vi "LPT-GUI-MIC-ver 5b.vi"() -> ()   [LabVIEW 2019]
uses:
  <vilib>/userDefined/High Color/IMAQdx.ctl
  LabView - DISB Eval SW 2.6/LabView - DISB Eval SW 2.6/Register name.ctl
  <vilib>/Utility/file.llb/Write Delimited Spreadsheet (DBL).vi
  <vilib>/vision/driver/NI_Vision_Acquisition_Software.lvlib
panel:
  in  "LED Resource (write)":refnum<visa-resource-name>="COM3"
  in  "Session In 2":T1="cam6"
  in  "Session In":T1="cam5"
  out "COMMAND1 READ 3":string="LED1 ON\r"
  out "AUT FOCUS STATUS 2":bool
  out "Position (um) 2":dbl(slide) min=0.0 max=100.0 step=0.01 scale=0.0..1500.0
  out "COMMAND 3":string="LED1 OFF"
  out "NUMBER 2":string
  out "Raw Data 2":sgl[](graph)
  out "power sum 2":sgl
  in  "#of steps 3":i32=200
  in  "STAGE START 2":i32
  in  "STAGE STOP 2":i32=20
  out "power sum":sgl
  out "Raw Data":sgl[](graph)
  in  "START CAM TAB":bool
  out "Camera STOP 2":bool
  out "COMMAND1 READ 2":string="LED1 ON\r"
  out "Position (um)":dbl(slide) min=0.0 max=100.0 step=0.01 scale=0.0..1500.0
  out "COMMAND 2":string="LED1 OFF"
  out "NUMBER":string
  in  "#of steps 2":i32=5
  in  "STAGE START":i32
  in  "STAGE STOP":i32=1500
  out "BOROSCOPE END":string
  out "Position (mm)":dbl(slide)=10.0 min=0.0 max=100.0 step=0.01 scale=0.0..20.0 scale format="%.2f"
  out "COMMAND1 READ":string="LED1 ON\r"
  in  "COMMAND 1":string="LED1 OFF"
  out "LASER \nFOCUSED":bool
  in  "INTERACTIVE CONTROLS":T2(radio)
  in  "LQComm resource name":refnum<visa-resource-name>="COM4"
  in  "Analysis Program":T3(radio)
  in  "LIBS Laser Frequency (Hz)":u16=10 min=10 max=1000
  in  "Auto Set\nLaser Frequency":bool
  in  "Acquisition Type":enum32{"RAMAN", "LIBS"}(radio)
  in  "Integration\n Time (ms)":i32=100
  in  "ID spectra":bool
  in  "Number of Scans \nto Auto Acquire":i32=2
  in  "AutoAcquire":bool=TRUE
  out "power setting from LQ":string="POWER=080\r\n"
  out "Power Out":dbl=0.4
  in  "Get Dark?":bool
  in  "Set Power (mW)":i32=80
  in  "Start":bool
  out "Camera STOP":bool
  in  "EXIT INTERACTIVE CONTROL":bool
  in  "ABORT  LOOP":bool
  out "Removed background":dbl[](graph)
  out "LIBS Dark Spectra":dbl[](graph)
  out "Dark Spectra":dbl[](graph)=[1870.0, 1885.0, 1880.0, 1896.0, 1901.0, 1906.0, 1893.0, 1873.0, 1869.0, 1877.0, 1867.0, 1828.0, 1817.0, 1812.0, 1819.0, 1837.0, 1828.0, 1798.0, 1797.0, 1809.0, 1800.0, 1781.0, 1773.0, 1752.0, 1749.0, 1759.0, 1771.0, 1780.0, 1783.0, 1757.0, 1759.0, 1773.0, 1764.0, 1750.0, 1783.0, 1813.0, 1852.0, 1868.0, 1849.0, 1845.0, 1844.0, 1863.0, 1853.0, 1841.0, 1791.0, 1771.0, 1777.0, 1785.0, 1821.0, 1881.0, 1909.0, 1926.0, 1925.0, 1929.0, 1912.0, 1898.0, 1903.0, 1901.0, 1897.0, 1865.0, 1874.0, 1897.0, 1919.0, 1905.0, 1901.0, 1919.0, 1947.0, 1919.0, 1887.0, 1877.0, 1837.0, 1807.0, 1823.0, 1855.0, 1871.0, 1847.0, 1823.0, 1842.0, 1887.0, 1906.0, 1925.0, 1945.0, 1924.0, 1919.0, 1919.0, 1906.0, 1897.0, 1865.0, 1817.0, 1801.0, 1809.0, 1797.0, 1818.0, 1860.0, 1853.0, 1819.0, 1768.0, 1758.0, 1741.0, 1732.0, 1717.0, 1725.0, 1734.0, 1713.0, 1695.0, 1707.0, 1727.0, 1743.0, 1759.0, 1788.0, 1802.0, 1775.0, 1772.0, 1780.0, 1801.0, 1819.0, 1813.0, 1817.0, 1823.0, 1844.0, 1851.0, 1805.0, 1809.0, 1842.0, 1845.0, 1853.0, 1837.0, 1846.0, 1837.0, 1853.0, 1862.0, 1881.0, 1901.0, 1874.0, 1861.0, 1892.0, 1876.0, 1872.0, 1855.0, 1846.0, 1860.0, 1861.0, 1887.0, 1887.0, 1883.0, 1897.0, 1897.0, 1903.0, 1911.0, 1901.0, 1880.0, 1871.0, 1855.0, 1879.0, 1860.0, 1871.0, 1880.0, 1879.0, 1858.0, 1855.0, 1837.0, 1837.0, 1823.0, 1828.0, 1807.0, 1821.0, 1882.0, 1890.0, 1893.0, 1860.0, 1832.0, 1812.0, 1813.0, 1842.0, 1852.0, 1849.0, 1851.0, 1835.0, 1849.0, 1885.0, 1924.0, 1930.0, 1930.0, 1925.0, 1892.0, 1897.0, 1903.0, 1900.0, 1912.0, 1917.0, 1946.0, 1947.0, 1927.0, 1896.0, 1881.0, 1896.0, 1874.0, 1873.0, 1876.0, 1898.0, 1899.0, 1885.0, 1892.0, 1897.0, 1896.0, 1896.0, 1878.0, 1870.0, 1860.0, 1853.0, 1867.0, 1855.0, 1839.0, 1839.0, 1849.0, 1853.0, 1846.0, 1829.0, 1817.0, 1828.0, 1823.0, 1860.0, 1881.0, 1863.0, 1885.0, 1860.0, 1833.0, 1846.0, 1832.0, 1844.0, 1813.0, 1815.0, 1837.0, 1833.0, 1837.0, 1828.0, 1829.0, 1844.0, 1840.0, 1849.0, 1844.0, 1812.0, 1815.0, 1801.0, 1814.0, 1815.0, 1837.0, 1832.0, 1840.0, 1812.0, 1797.0, 1815.0, 1862.0, 1899.0, 1906.0, 1905.0, 1885.0, 1868.0, 1861.0, 1845.0, 1832.0, 1797.0, 1803.0, 1791.0, 1791.0, 1784.0, 1801.0, 1786.0, 1768.0, 1765.0, 1759.0, 1745.0, 1743.0, 1774.0, 1813.0, 1820.0, 1855.0, 1881.0, 1881.0, 1887.0, 1876.0, 1870.0, 1864.0, 1897.0, 1897.0, 1887.0, 1873.0, 1853.0, 1833.0, 1807.0, 1802.0, 1791.0, 1823.0, 1828.0, 1812.0, 1850.0, 1853.0, 1846.0, 1839.0, 1837.0, 1852.0, 1849.0, 1828.0, 1848.0, 1864.0, 1860.0, 1864.0, 1846.0, 1829.0, 1837.0, 1835.0, 1819.0, 1807.0, 1812.0, 1805.0, 1789.0, 1798.0, 1802.0, 1818.0, 1783.0, 1796.0, 1804.0, 1837.0, 1876.0, 1935.0, 1994.0, 2007.0, 1969.0, 1961.0, 1938.0, 1917.0, 1908.0, 1901.0, 1885.0, 1911.0, 1930.0, 1929.0, 1945.0, 1919.0, 1899.0, 1870.0, 1855.0, 1825.0, 1814.0, 1817.0, 1797.0, 1803.0, 1791.0, 1789.0, 1768.0, 1734.0, 1757.0, 1757.0, 1737.0, 1752.0, 1773.0, 1768.0, 1761.0, 1759.0, 1784.0, 1783.0, 1803.0, 1791.0, 1791.0, 1796.0, 1791.0, 1781.0, 1773.0, 1761.0, 1780.0, 1791.0, 1780.0, 1773.0, 1759.0, 1757.0, 1769.0, 1773.0, 1768.0, 1780.0, 1780.0, 1782.0, 1807.0, 1805.0, 1789.0, 1807.0, 1836.0, 1823.0, 1839.0, 1873.0, 1873.0, 1893.0, 1892.0, 1868.0, 1876.0, 1887.0, 1896.0, 1899.0, 1892.0, 1867.0, 1851.0, 1848.0, 1839.0, 1865.0, 1866.0, 1849.0, 1834.0, 1839.0, 1862.0, 1861.0, 1851.0, 1839.0, 1849.0, 1847.0, 1828.0, 1789.0, 1769.0, 1787.0, 1779.0, 1797.0, 1816.0, 1846.0, 1855.0, 1855.0, 1863.0, 1869.0, 1885.0, 1892.0, 1901.0, 1946.0, 1913.0, 1880.0, 1896.0, 1901.0, 1877.0, 1881.0, 1878.0, 1855.0, 1845.0, 1832.0, 1799.0, 1769.0, 1757.0, 1781.0, 1762.0, 1735.0, 1714.0, 1733.0, 1757.0, 1773.0, 1773.0, 1783.0, 1778.0, 1768.0, 1764.0, 1765.0, 1753.0, 1738.0, 1759.0, 1781.0, 1789.0, 1800.0, 1799.0, 1796.0, 1785.0, 1771.0, 1727.0, 1700.0, 1723.0, 1711.0, 1716.0, 1738.0, 1773.0, 1781.0, 1769.0, 1778.0, 1768.0, 1771.0, 1775.0, 1781.0, 1768.0, 1744.0, 1739.0, 1732.0, 1716.0, 1695.0, 1689.0, 1695.0, 1679.0, 1695.0, 1692.0, 1717.0, 1718.0, 1721.0, 1695.0, 1679.0, 1677.0, 1675.0, 1678.0, 1679.0, 1682.0, 1689.0, 1684.0, 1711.0, 1711.0, 1721.0, 1727.0, 1727.0, 1723.0, 1707.0, 1732.0, 1721.0, 1724.0, 1700.0, 1692.0, 1685.0, 1693.0, 1695.0, 1705.0, 1694.0, 1700.0, 1722.0, 1714.0, 1719.0, 1723.0, 1711.0, 1721.0, 1746.0, 1775.0, 1756.0, 1704.0, 1692.0, 1721.0, 1725.0, 1718.0, 1712.0, 1725.0, 1732.0, 1741.0, 1745.0, 1773.0, 1784.0, 1782.0, 1785.0, 1800.0, 1800.0, 1785.0, 1757.0, 1759.0, 1718.0, 1725.0, 1725.0, 1736.0, 1770.0, 1802.0, 1808.0, 1801.0, 1809.0, 1812.0, 1794.0, 1823.0, 1842.0, 1839.0, 1849.0, 1823.0, 1832.0, 1823.0, 1801.0, 1812.0, 1832.0, 1823.0, 1810.0, 1810.0, 1796.0, 1816.0, 1797.0, 1853.0, 1871.0, 1883.0, 1887.0, 1902.0, 1884.0, 1869.0, 1853.0, 1832.0, 1823.0, 1812.0, 1821.0, 1823.0, 1832.0, 1821.0, 1823.0, 1809.0, 1784.0, 1752.0, 1732.0, 1727.0, 1721.0, 1709.0, 1735.0, 1727.0, 1725.0, 1707.0, 1698.0, 1682.0, 1689.0, 1714.0, 1716.0, 1707.0, 1709.0, 1714.0, 1725.0, 1727.0, 1738.0, 1725.0, 1741.0, 1739.0, 1701.0, 1733.0, 1727.0, 1717.0, 1718.0, 1752.0, 1775.0, 1775.0, 1784.0, 1802.0, 1771.0, 1759.0, 1750.0, 1724.0, 1721.0, 1711.0, 1689.0, 1677.0, 1666.0, 1686.0, 1698.0, 1711.0, 1750.0, 1741.0, 1756.0, 1771.0, 1768.0, 1787.0, 1796.0, 1807.0, 1790.0, 1809.0, 1842.0, 1832.0, 1807.0, 1805.0, 1805.0, 1764.0, 1789.0, 1785.0, 1669.0, 1625.0, 1631.0, 1637.0, 1642.0, 1599.0, 1605.0, 1579.0, 1592.0, 1576.0, 1590.0, 1604.0, 1615.0, 1659.0, 1672.0, 1669.0, 1689.0, 1672.0, 1672.0, 1701.0, 1716.0, 1741.0, 1730.0, 1719.0, 1711.0, 1695.0, 1706.0, 1721.0, 1770.0, 1796.0, 1797.0, 1768.0, 1765.0, 1781.0, 1765.0, 1759.0, 1749.0, 1781.0, 1786.0, 1804.0, 1796.0, 1777.0, 1768.0, 1772.0, 1778.0, 1821.0, 1821.0, 1823.0, 1837.0, 1845.0, 1829.0, 1849.0, 1833.0, 1832.0, 1797.0, 1771.0, 1764.0, 1791.0, 1786.0, 1764.0, 1743.0, 1730.0, 1752.0, 1746.0, 1741.0, 1741.0, 1748.0, 1757.0, 1784.0, 1775.0, 1777.0, 1796.0, 1810.0, 1799.0, 1814.0, 1768.0, 1773.0, 1780.0, 1765.0, 1764.0, 1769.0, 1748.0, 1732.0, 1709.0, 1706.0, 1695.0, 1679.0, 1675.0, 1669.0, 1679.0, 1707.0, 1721.0, 1711.0, 1704.0, 1701.0, 1700.0, 1695.0, 1695.0, 1668.0, 1692.0, 1711.0, 1725.0, 1716.0, 1693.0, 1700.0, 1720.0, 1704.0, 1711.0, 1716.0, 1725.0, 1721.0, 1706.0, 1700.0, 1706.0, 1717.0, 1732.0, 1717.0, 1721.0, 1695.0, 1695.0, 1698.0, 1688.0, 1689.0, 1691.0, 1687.0, 1709.0, 1717.0, 1732.0, 1725.0, 1668.0, 1672.0, 1673.0, 1681.0, 1688.0, 1707.0, 1725.0, 1739.0, 1716.0, 1641.0, 1636.0, 1642.0, 1655.0, 1663.0, 1675.0, 1675.0, 1700.0, 1730.0, 1764.0, 1803.0, 1816.0, 1820.0, 1807.0, 1791.0, 1759.0, 1753.0, 1761.0, 1759.0, 1753.0, 1744.0, 1775.0, 1781.0, 1768.0, 1753.0, 1741.0, 1721.0, 1725.0, 1743.0, 1748.0, 1747.0, 1771.0, 1775.0, 1771.0, 1756.0, 1753.0, 1709.0, 1716.0, 1704.0, 1734.0, 1737.0, 1725.0, 1721.0, 1724.0, 1716.0, 1732.0, 1744.0, 1775.0, 1751.0, 1706.0, 1704.0, 1716.0, 1709.0, 1717.0, 1741.0, 1761.0, 1764.0, 1781.0, 1791.0, 1764.0, 1746.0, 1732.0, 1734.0, 1727.0, 1716.0, 1700.0, 1686.0, 1684.0, 1686.0, 1707.0, 1732.0, 1727.0, 1738.0, 1716.0, 1705.0, 1709.0, 1707.0, 1700.0, 1698.0, 1698.0, 1716.0, 1723.0, 1705.0, 1717.0, 1689.0, 1690.0, 1687.0, 1684.0, 1719.0, 1717.0, 1714.0, 1690.0, 1668.0, 1663.0, 1675.0, 1677.0, 1684.0, 1673.0, 1668.0, 1679.0, 1695.0, 1706.0, 1735.0, 1748.0, 1747.0, 1759.0, 1764.0, 1757.0, 1732.0, 1750.0, 1781.0, 1764.0, 1764.0, 1749.0, 1754.0, 1756.0, 1741.0, 1739.0, 1741.0, 1714.0, 1733.0, 1762.0, 1759.0, 1768.0, 1775.0, 1768.0, 1759.0, 1768.0, 1750.0, 1739.0, 1757.0, 1757.0, 1727.0, 1748.0, 1723.0, 1725.0, 1709.0, 1709.0, 1709.0, 1731.0, 1734.0, 1748.0, 1759.0, 1757.0, 1759.0, 1752.0, 1741.0, 1755.0, 1787.0, 1791.0, 1820.0, 1840.0, 1860.0, 1873.0, 1874.0, 1865.0, 1876.0, 1876.0, 1844.0, 1844.0, 1849.0, 1862.0, 1832.0, 1828.0, 1842.0, 1832.0, 1796.0, 1788.0, 1751.0, 1764.0, 1756.0, 1746.0, 1739.0, 1733.0, 1726.0, 1705.0, 1700.0, 1723.0, 1725.0, 1725.0, 1739.0, 1759.0, 1777.0, 1771.0, 1759.0, 1771.0, 1765.0, 1753.0, 1725.0, 1684.0, 1647.0, 1636.0, 1652.0, 1657.0, 1669.0, 1672.0, 1677.0, 1653.0, 1672.0, 1657.0, 1661.0, 1660.0, 1676.0, 1704.0, 1707.0, 1729.0, 1757.0, 1796.0, 1797.0, 1802.0, 1797.0, 1807.0, 1844.0, 1835.0, 1794.0, 1791.0, 1796.0, 1801.0, 1789.0, 1791.0, 1782.0, 1768.0, 1739.0, 1723.0, 1736.0, 1732.0, 1737.0, 1733.0, 1727.0, 1707.0, 1677.0, 1695.0, 1704.0, 1714.0, 1690.0, 1657.0, 1661.0, 1669.0, 1656.0, 1652.0, 1611.0, 1595.0, 1549.0, 1562.0, 1596.0, 1610.0, 1573.0, 1576.0, 1577.0, 1567.0, 1573.0, 1605.0, 1592.0, 1622.0, 1621.0, 1609.0, 1599.0, 1606.0, 1581.0, 1565.0, 1567.0, 1589.0, 1610.0, 1607.0, 1608.0, 1643.0, 1647.0, 1668.0, 1691.0, 1675.0, 1641.0, 1647.0, 1640.0, 1622.0, 1621.0, 1588.0, 1602.0, 1622.0, 1611.0, 1599.0, 1602.0, 1640.0, 1643.0, 1647.0, 1629.0, 1577.0, 1547.0, 1554.0, 1551.0, 1540.0, 1561.0, 1561.0, 1576.0, 1614.0, 1674.0, 1707.0, 1717.0, 1736.0, 1735.0, 1743.0, 1738.0, 1727.0, 1735.0, 1721.0, 1721.0, 1687.0, 1707.0, 1709.0, 1748.0, 1743.0, 1743.0, 1753.0, 1769.0, 1759.0, 1765.0, 1737.0, 1727.0, 1711.0, 1679.0, 1672.0, 1686.0, 1672.0, 1668.0, 1660.0, 1645.0, 1669.0, 1688.0, 1685.0, 1679.0, 1721.0, 1739.0, 1712.0, 1681.0, 1650.0, 1653.0, 1661.0, 1663.0, 1663.0, 1668.0, 1672.0, 1704.0, 1714.0, 1721.0, 1718.0, 1814.0, 1797.0, 1759.0, 1754.0, 1743.0, 1762.0, 1748.0, 1768.0, 1741.0, 1690.0, 1707.0, 1717.0, 1739.0, 1768.0, 1727.0, 1682.0, 1650.0, 1681.0, 1701.0, 1727.0, 1695.0, 1676.0, 1673.0, 1669.0, 1677.0, 1663.0, 1674.0, 1690.0, 1687.0, 1668.0, 1690.0, 1725.0, 1689.0, 1647.0, 1627.0, 1615.0, 1647.0, 1656.0, 1631.0, 1625.0, 1618.0, 1609.0, 1608.0, 1636.0, 1674.0, 1720.0, 1738.0, 1745.0, 1736.0, 1738.0, 1762.0, 1781.0, 1776.0, 1794.0, 1798.0, 1757.0, 1741.0, 1717.0, 1711.0, 1725.0, 1727.0, 1732.0, 1730.0, 1701.0, 1700.0, 1657.0, 1652.0, 1668.0, 1653.0, 1621.0, 1629.0, 1611.0, 1615.0, 1608.0, 1583.0, 1599.0, 1636.0, 1668.0, 1684.0, 1705.0, 1701.0, 1725.0, 1752.0, 1746.0, 1749.0, 1727.0, 1755.0, 1746.0, 1749.0, 1764.0, 1752.0, 1739.0, 1768.0, 1757.0, 1711.0, 1677.0, 1657.0, 1653.0, 1661.0, 1647.0, 1618.0, 1620.0, 1649.0, 1675.0, 1668.0, 1672.0, 1679.0, 1656.0, 1669.0, 1674.0, 1700.0, 1705.0, 1704.0, 1700.0, 1705.0, 1718.0, 1711.0, 1705.0, 1701.0, 1718.0, 1713.0, 1736.0, 1752.0, 1748.0, 1732.0, 1750.0, 1765.0, 1741.0, 1723.0, 1725.0, 1705.0, 1676.0, 1641.0, 1636.0, 1631.0, 1631.0, 1656.0, 1663.0, 1666.0, 1668.0, 1669.0, 1629.0, 1647.0, 1610.0, 1551.0, 1494.0, 1483.0, 1465.0, 1476.0, 1487.0, 1512.0, 1553.0, 1573.0, 1556.0, 1501.0, 1503.0, 1531.0, 1567.0, 1624.0, 1663.0, 1661.0, 1657.0, 1645.0, 1616.0, 1621.0, 1594.0, 1529.0, 1503.0, 1490.0, 1476.0, 1501.0, 1501.0, 1517.0, 1527.0, 1558.0, 1567.0, 1586.0, 1556.0, 1547.0, 1548.0, 1551.0, 1497.0, 1439.0, 1428.0, 1459.0, 1516.0, 1563.0, 1558.0, 1609.0, 1657.0, 1693.0, 1734.0, 1753.0, 1765.0, 1773.0, 1796.0, 1800.0, 1815.0, 1821.0, 1851.0, 1855.0, 1844.0, 1844.0, 1846.0, 1850.0, 1833.0, 1786.0, 1791.0, 1791.0, 1789.0, 1798.0, 1797.0, 1802.0, 1809.0, 1819.0, 1820.0, 1816.0, 1796.0, 1804.0, 1804.0, 1786.0, 1794.0, 1753.0, 1764.0, 1800.0, 1811.0, 1809.0, 1816.0, 1785.0, 1765.0, 1735.0, 1687.0, 1672.0, 1661.0, 1621.0, 1583.0, 1482.0, 1444.0, 1451.0, 1471.0, 1500.0, 1541.0, 1530.0, 1541.0, 1540.0, 1581.0, 1605.0, 1649.0, 1659.0, 1660.0, 1654.0, 1672.0, 1668.0, 1691.0, 1692.0, 1693.0, 1672.0, 1674.0, 1693.0, 1707.0, 1735.0, 1759.0, 1758.0, 1752.0, 1759.0, 1763.0, 1764.0, 1757.0, 1741.0, 1727.0, 1727.0, 1720.0, 1738.0, 1733.0, 1735.0, 1725.0, 1743.0, 1746.0, 1753.0, 1752.0, 1750.0, 1738.0, 1755.0, 1746.0, 1764.0, 1787.0, 1775.0, 1748.0, 1725.0, 1725.0, 1759.0, 1775.0, 1791.0, 1804.0, 1823.0, 1842.0, 1839.0, 1846.0, 1807.0, 1812.0, 1835.0, 1819.0, 1837.0, 1799.0, 1769.0, 1765.0, 1759.0, 1781.0, 1768.0, 1727.0, 1689.0, 1672.0, 1636.0, 1629.0, 1629.0, 1647.0, 1645.0, 1641.0, 1640.0, 1658.0, 1640.0, 1642.0, 1645.0, 1672.0, 1700.0, 1701.0, 1688.0, 1709.0, 1727.0, 1732.0, 1759.0, 1754.0, 1765.0, 1746.0, 1727.0, 1725.0, 1759.0, 1752.0, 1753.0, 1768.0, 1759.0, 1764.0, 1759.0, 1773.0, 1794.0, 1796.0, 1791.0, 1812.0, 1805.0, 1810.0, 1801.0, 1791.0, 1782.0, 1787.0, 1775.0, 1775.0, 1775.0, 1780.0, 1783.0, 1807.0, 1815.0, 1821.0, 1800.0, 1823.0, 1819.0, 1801.0, 1779.0, 1773.0, 1780.0, 1788.0, 1804.0, 1800.0, 1789.0, 1757.0, 1743.0, 1727.0, 1721.0, 1732.0, 1720.0, 1681.0, 1681.0, 1701.0, 1684.0, 1650.0, 1645.0, 1656.0, 1684.0, 1686.0, 1677.0, 1691.0, 1685.0, 1700.0, 1721.0, 1741.0, 1758.0, 1749.0, 1733.0, 1695.0, 1701.0, 1687.0, 1712.0, 1721.0, 1738.0, 1759.0, 1796.0, 1823.0, 1849.0, 1860.0, 1868.0, 1855.0, 1848.0, 1855.0, 1844.0, 1809.0, 1810.0, 1832.0, 1807.0, 1800.0, 1829.0, 1837.0, 1823.0, 1805.0, 1828.0, 1848.0, 1855.0, 1838.0, 1807.0, 1804.0, 1802.0, 1806.0, 1823.0, 1807.0, 1807.0, 1816.0, 1844.0, 1862.0, 1879.0, 1882.0, 1877.0, 1875.0, 1897.0, 1855.0, 1837.0, 1835.0, 1817.0, 1810.0, 1789.0, 1751.0, 1741.0, 1723.0, 1722.0, 1718.0, 1752.0, 1773.0, 1768.0, 1781.0, 1739.0, 1709.0, 1693.0, 1709.0, 1722.0, 1727.0, 1724.0, 1749.0, 1725.0, 1748.0, 1758.0, 1769.0, 1778.0, 1771.0, 1770.0, 1745.0, 1736.0, 1771.0, 1768.0, 1748.0, 1756.0, 1773.0, 1748.0, 1754.0, 1772.0, 1804.0, 1803.0, 1805.0, 1768.0, 1750.0, 1764.0, 1741.0, 1748.0, 1727.0, 1707.0, 1707.0, 1737.0, 1721.0, 1717.0, 1722.0, 1720.0, 1734.0, 1750.0, 1725.0, 1725.0, 1736.0, 1691.0, 1681.0, 1689.0, 1677.0, 1675.0, 1707.0, 1712.0, 1704.0, 1684.0, 1679.0, 1677.0, 1683.0, 1663.0, 1636.0, 1640.0, 1640.0, 1657.0, 1669.0, 1677.0, 1704.0, 1727.0, 1769.0, 1741.0, 1749.0, 1759.0, 1757.0, 1762.0, 1750.0, 1749.0, 1759.0, 1759.0, 1775.0, 1773.0, 1823.0, 1815.0, 1807.0, 1821.0, 1813.0, 1805.0, 1817.0, 1813.0, 1821.0, 1807.0, 1803.0, 1805.0, 1821.0, 1828.0, 1817.0, 1805.0, 1802.0, 1791.0, 1776.0, 1768.0, 1770.0, 1755.0, 1738.0, 1764.0, 1757.0, 1751.0, 1759.0, 1762.0, 1786.0, 1771.0, 1775.0, 1801.0, 1807.0, 1797.0, 1786.0, 1855.0, 1879.0, 1878.0, 1852.0, 1834.0, 1845.0, 1849.0, 1869.0, 1865.0, 1855.0, 1885.0, 1885.0, 1860.0, 1812.0, 1803.0, 1790.0, 1784.0, 1773.0, 1769.0, 1751.0, 1739.0, 1721.0, 1749.0, 1738.0, 1742.0, 1743.0, 1718.0, 1687.0, 1685.0, 1700.0, 1724.0, 1753.0, 1746.0, 1745.0, 1781.0, 1810.0, 1812.0, 1823.0, 1805.0, 1821.0, 1820.0, 1790.0, 1780.0, 1791.0, 1798.0, 1804.0, 1837.0, 1869.0, 1871.0, 1884.0, 1887.0, 1887.0, 1906.0, 1906.0, 1917.0, 1897.0, 1870.0, 1892.0, 1885.0, 1866.0, 1855.0, 1861.0, 1840.0, 1849.0, 1860.0, 1853.0, 1823.0, 1832.0, 1855.0, 1853.0, 1853.0, 1836.0, 1832.0, 1829.0, 1835.0, 1819.0, 1805.0, 1797.0, 1770.0, 1768.0, 1769.0, 1796.0, 1759.0, 1766.0, 1780.0, 1822.0, 1839.0, 1876.0, 1892.0, 1878.0, 1865.0, 1846.0, 1844.0, 1817.0, 1828.0, 1821.0, 1807.0, 1801.0, 1771.0, 1807.0, 1783.0, 1789.0, 1778.0, 1787.0, 1780.0, 1765.0, 1768.0, 1773.0, 1777.0, 1773.0, 1775.0, 1781.0, 1771.0, 1777.0, 1789.0, 1802.0, 1818.0, 1823.0, 1805.0, 1804.0, 1801.0, 1802.0, 1828.0, 1791.0, 1784.0, 1765.0, 1756.0, 1748.0, 1727.0, 1712.0, 1714.0, 1749.0, 1775.0, 1789.0, 1780.0, 1781.0, 1756.0, 1755.0, 1759.0, 1771.0, 1759.0, 1755.0, 1748.0, 1748.0, 1743.0, 1708.0, 1707.0, 1704.0, 1672.0, 1650.0, 1631.0, 1650.0, 1652.0, 1652.0, 1660.0, 1669.0, 1685.0, 1713.0, 1711.0, 1692.0, 1734.0, 1753.0, 1753.0, 1759.0, 1727.0, 1736.0, 1771.0, 1786.0, 1789.0, 1764.0, 1732.0, 1736.0, 1737.0, 1736.0, 1736.0, 1761.0, 1768.0, 1759.0, 1768.0, 1748.0, 1716.0, 1723.0, 1733.0, 1725.0, 1727.0, 1738.0, 1727.0, 1732.0, 1735.0, 1756.0, 1791.0, 1791.0, 1796.0, 1832.0, 1865.0, 1885.0, 1884.0, 1885.0, 1873.0, 1878.0, 1855.0, 1821.0, 1812.0, 1819.0, 1823.0, 1809.0, 1816.0, 1813.0, 1808.0, 1803.0, 1807.0, 1795.0, 1805.0, 1823.0, 1821.0, 1839.0, 1844.0, 1861.0, 1861.0, 1892.0, 1913.0, 1919.0, 1885.0, 1885.0, 1885.0, 1869.0, 1861.0, 1871.0, 1885.0, 1930.0, 1929.0, 1883.0, 1887.0, 1877.0, 1865.0, 1855.0, 1851.0, 1835.0, 1821.0, 1808.0, 1759.0, 1773.0, 1783.0, 1773.0, 1786.0, 1781.0, 1768.0, 1776.0, 1757.0, 1785.0, 1802.0, 1797.0, 1796.0, 1805.0, 1808.0, 1800.0, 1798.0, 1821.0, 1832.0, 1799.0, 1795.0, 1800.0, 1813.0, 1823.0, 1842.0, 1887.0, 1909.0, 1909.0, 1908.0, 1893.0, 1865.0, 1855.0, 1832.0, 1828.0, 1805.0, 1819.0, 1832.0, 1818.0, 1820.0, 1805.0, 1784.0, 1780.0, 1785.0, 1783.0, 1789.0, 1752.0, 1740.0, 1711.0, 1721.0, 1736.0, 1732.0, 1727.0, 1738.0, 1756.0, 1804.0, 1817.0, 1832.0, 1846.0, 1853.0, 1833.0, 1817.0, 1807.0, 1776.0, 1775.0, 1757.0, 1750.0, 1745.0, 1771.0, 1778.0, 1800.0, 1805.0, 1781.0, 1797.0, 1796.0, 1789.0, 1778.0, 1759.0, 1744.0, 1751.0, 1755.0, 1762.0, 1737.0, 1725.0, 1746.0, 1769.0, 1809.0, 1815.0, 1813.0, 1786.0, 1769.0, 1768.0, 1770.0, 1764.0, 1765.0, 1768.0, 1755.0, 1736.0, 1759.0, 0.0, 0.0, 0.0, 0.0, 0.0]
  out "STATUS":string="INITIALIZING LIBS"
  in  "STAGE STOP A":i32=19 min=10 max=19 format="%.2f"
  in  "STAGE START A":i32=1 min=1 max=10 format="%.2f"
  in  "#of steps A":i32=18 min=2 max=100
  in  "AUT FOCUS":bool
  out "Spectrum":cluster{dbl[], "Dark Array":dbl[]}(graph)
  out "msPerClock":dbl
  in  "SPI clock frequency [Hz]":u32
  in  "*Cal coef":dbl[](array[numeric])=[0.0] format="%.7e"
  in  "*Wavelength axis":dbl[](array[numeric]) format="%.7e"
  in  "Pixel axis":u16[](array[numeric])
  out "Dark spectrum":dbl[](array[numeric])
  out "Ref spectrum":dbl[](array[numeric])
  in  "*Production mode":u16 format="%x"
  in  "*Sensor ctrl":u16
  in  "Skipping start read buffer":u16 max=4096
  in  "Skipping end read buffer":u16=17 min=17 max=4096
  in  "*Last pixel of interest":u16=17 min=17 max=4096
  in  "*First pixel of interest":u16 max=4096
  out "*FW - Reserved":u16
  out "*FW - Variant":u16
  out "*FW - Revision":u16
  out "*Spectrometer SN":u16
  out "Average in progress":bool
  in  "*Auto trig":bool=TRUE
  in  "*Averaging in HW":u16=1
  in  "*Data ready threshold":u16=1
  in  "*MPP mode change":u16
  out "Debug":u16
  out "*ADC offset [counts]":u16
  out "*ADC gain [counts]":u16
  out "Trigger delay MSB":u16
  out "Trigger delay LSB":u16
  out "Pixels ready":u16
  out "*Temperature  [counts] \n(12 bit ADC)":dbl
  out "Sensor exp time MSB":u16
  out "Sensor exp time LSB":u16
  out "*Calib data chars":u16
  out "*Pixels per image":u16
  out "*Detector type":u16
  out "*FW version":u16
  out "*HW version":u16
  out "*PCB SN":u16
  in  "Zero Dark LIBS":dbl[](array[numeric])
  in  "Data\\Dark":bool
  out "MaxPosition":dbl=500.0 format="%#_2f"
  out "max value":sgl=3651732.0
  in  "Zero Dark":dbl[](array[numeric])
  in  "Channel Settings":T4(array[cluster])=[{"Integration Time (msec)"=80, "Xtrate"=1, "Averaging"=5, "Smoothing"=4, "C1"=0.0, "C2"=0.0, "C3"=0.0, "C4"=0.0, "Digitizer Bits"=enum."12"}, {"Integration Time (msec)"=80, "Xtrate"=1, "Averaging"=5, "Smoothing"=4, "C1"=0.0, "C2"=0.0, "C3"=0.0, "C4"=0.0, "Digitizer Bits"=enum."12"}, {"Integration Time (msec)"=80, "Xtrate"=1, "Averaging"=5, "Smoothing"=4, "C1"=0.0, "C2"=0.0, "C3"=0.0, "C4"=0.0, "Digitizer Bits"=enum."12"}, {"Integration Time (msec)"=80, "Xtrate"=1, "Averaging"=5, "Smoothing"=4, "C1"=0.0, "C2"=0.0, "C3"=0.0, "C4"=0.0, "Digitizer Bits"=enum."12"}, {"Integration Time (msec)"=80, "Xtrate"=1, "Averaging"=5, "Smoothing"=4, "C1"=0.0, "C2"=0.0, "C3"=0.0, "C4"=0.0, "Digitizer Bits"=enum."12"}, {"Integration Time (msec)"=80, "Xtrate"=1, "Averaging"=5, "Smoothing"=4, "C1"=0.0, "C2"=0.0, "C3"=0.0, "C4"=0.0, "Digitizer Bits"=enum."12"}, {"Integration Time (msec)"=80, "Xtrate"=1, "Averaging"=5, "Smoothing"=4, "C1"=0.0, "C2"=0.0, "C3"=0.0, "C4"=0.0, "Digitizer Bits"=enum."12"}, {"Integration Time (msec)"=80, "Xtrate"=1, "Averaging"=5, "Smoothing"=4, "C1"=0.0, "C2"=0.0, "C3"=0.0, "C4"=0.0, "Digitizer Bits"=enum."12"}] caption="Spectrometer Configs" {"C4" format="%#.15f"; "C3" format="%#.15f"; "C2" format="%#.15f"; "C1" format="%#.15f"; "Smoothing" min=0 max=4 step=1; "Averaging" min=1 max=10000 step=1; "Xtrate" min=1 max=3; "Integration Time (msec)" min=1 max=2000}
  out "output\ncluster":T5={"Integration Time (ms)"=80, "Digitizer Clock Rate Setting"=3, "Number of Scans to Average"=1, "Optical Smoothing Level"=0, 0.096038248763, 3.43035e-07, -1.607e-09, -1.607e-09, 12}
  in  "RAMAN Spectometer\n Parameters":T6={"Integration Time (ms)"=80, "Digitizer Clock Rate Setting"=3, "Number of Scans to Average"=1, "Optical Smoothing Level"=0, "C1"=0.096038248763, "C2"=3.43035e-07, "C3"=536.3, "C4"=-1.607e-09, 12}
  in  "Tab Control":enum32{"Visible", "Fluorescence"}(tab)
  out "Visible Image":T7(plugin-control)
  out "Fluorescence Image":T7(plugin-control)
  in  "MOVE SPECTROMETER":bool
  out "AUT FOCUS STATUS":bool
  in  "Set End Position (um)":dbl(slide) scale=0.0..1500.0
  out "LED 2 STATUS":bool
  in  "LED 2":bool
  in  "LED 1":bool
  out "LED 1 STATUS":bool
  # "Laser and Plasma RAMAN/LIBS Acquisition Software"
  # "INITIAL SETTINGS"
  # "Raman Laser Settings"
  # "LIBS Laser Settings"
  # "LQC"
  # "LED"
  # "AUTO FOCUS SETTINGS"
  # "AUTO FOCUS RESULTS"
  # "V5b"
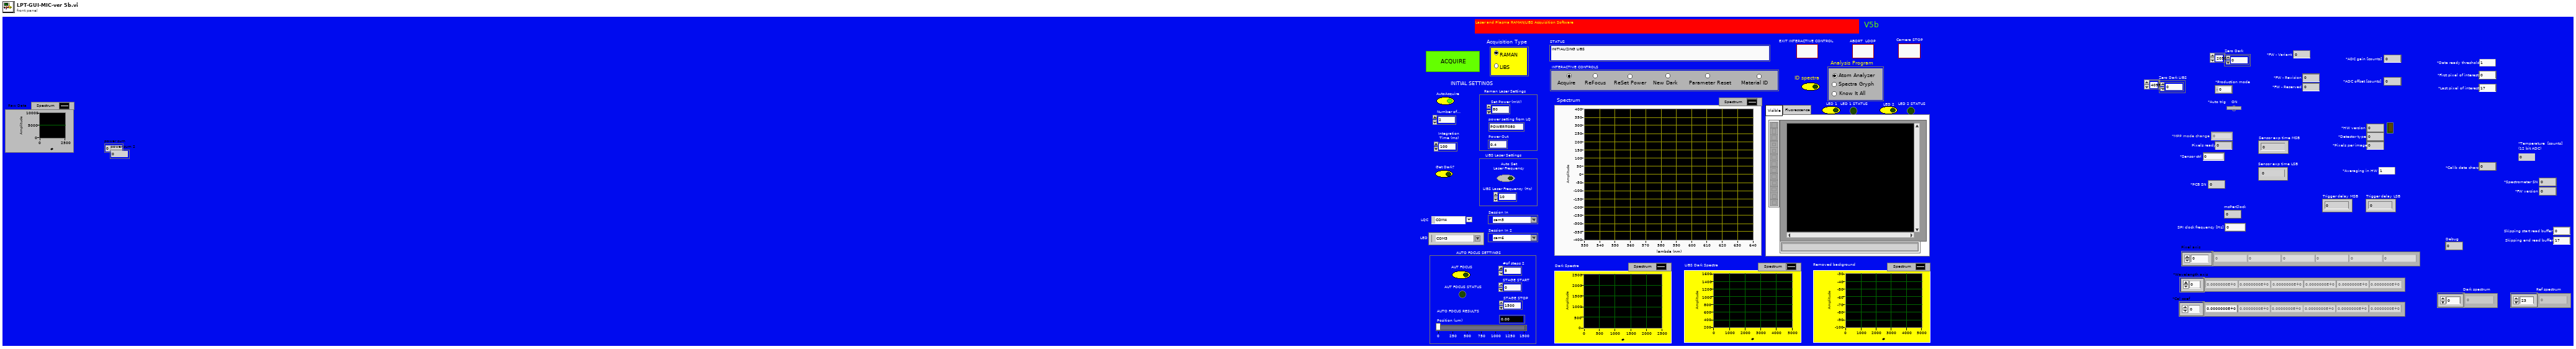
[diagram p1: front panel]
types:
  T1 = typedef "IMAQdx.ctl" = refnum<k21>
  T2 = enum32{"Acquire", "ReFocus", "ReSet Power", "New Dark", "Parameter Reset", "Material ID", "Do Nothing"}
  T3 = enum32{"Atom Analyzer", "Spectra Gryph", "Know It All"}
  T4 = cluster{"Integration Time (msec)":i32, "Xtrate":i32, "Averaging":i32, "Smoothing":i32, "C1":dbl, "C2":dbl, "C3":dbl, "C4":dbl, "Digitizer Bits":enum8{"12", "14", "16"}}[]
  T5 = cluster{"Integration Time (ms)":i32, "Digitizer Clock Rate Setting":i32, "Number of Scans to Average":i32, "Optical Smoothing Level":i32, dbl, dbl, dbl, dbl, i32}
  T6 = typedef "Control 1.ctl" = cluster{"Integration Time (ms)":i32, "Digitizer Clock Rate Setting":i32, "Number of Scans to Average":i32, "Optical Smoothing Level":i32, "C1":dbl, "C2":dbl, "C3":dbl, "C4":dbl, i32}
  T7 = typedef "IMAQ Image.ctl" = refnum<image>
  T8 = typedef "Register name.ctl" = enum8{"Serial number", "HW version", "FW version", "Detector type", "Pixel per image", "Calib data chars", "Calib data", "Sensor ctrl", "Sensor exp time LSB", "Sensor exp time MSB", "Temperature", "Pixel ready", "Trigger delay LSB", "Trigger delay MSB", "ADC PGA", "ADC offset", "Permanent storage", "MPP mode change", "DATA READY THRESHOLD", "IMAGES_TO_AVERAGE", "AVG_CONTROL", "SPECTROMETER SN", "SKIPPING_START", "SKIPPING_END", "debug", "Production mode"}
  T9 = enum8{"Enabled", "Disabled", "Disabled and Grayed Out"}
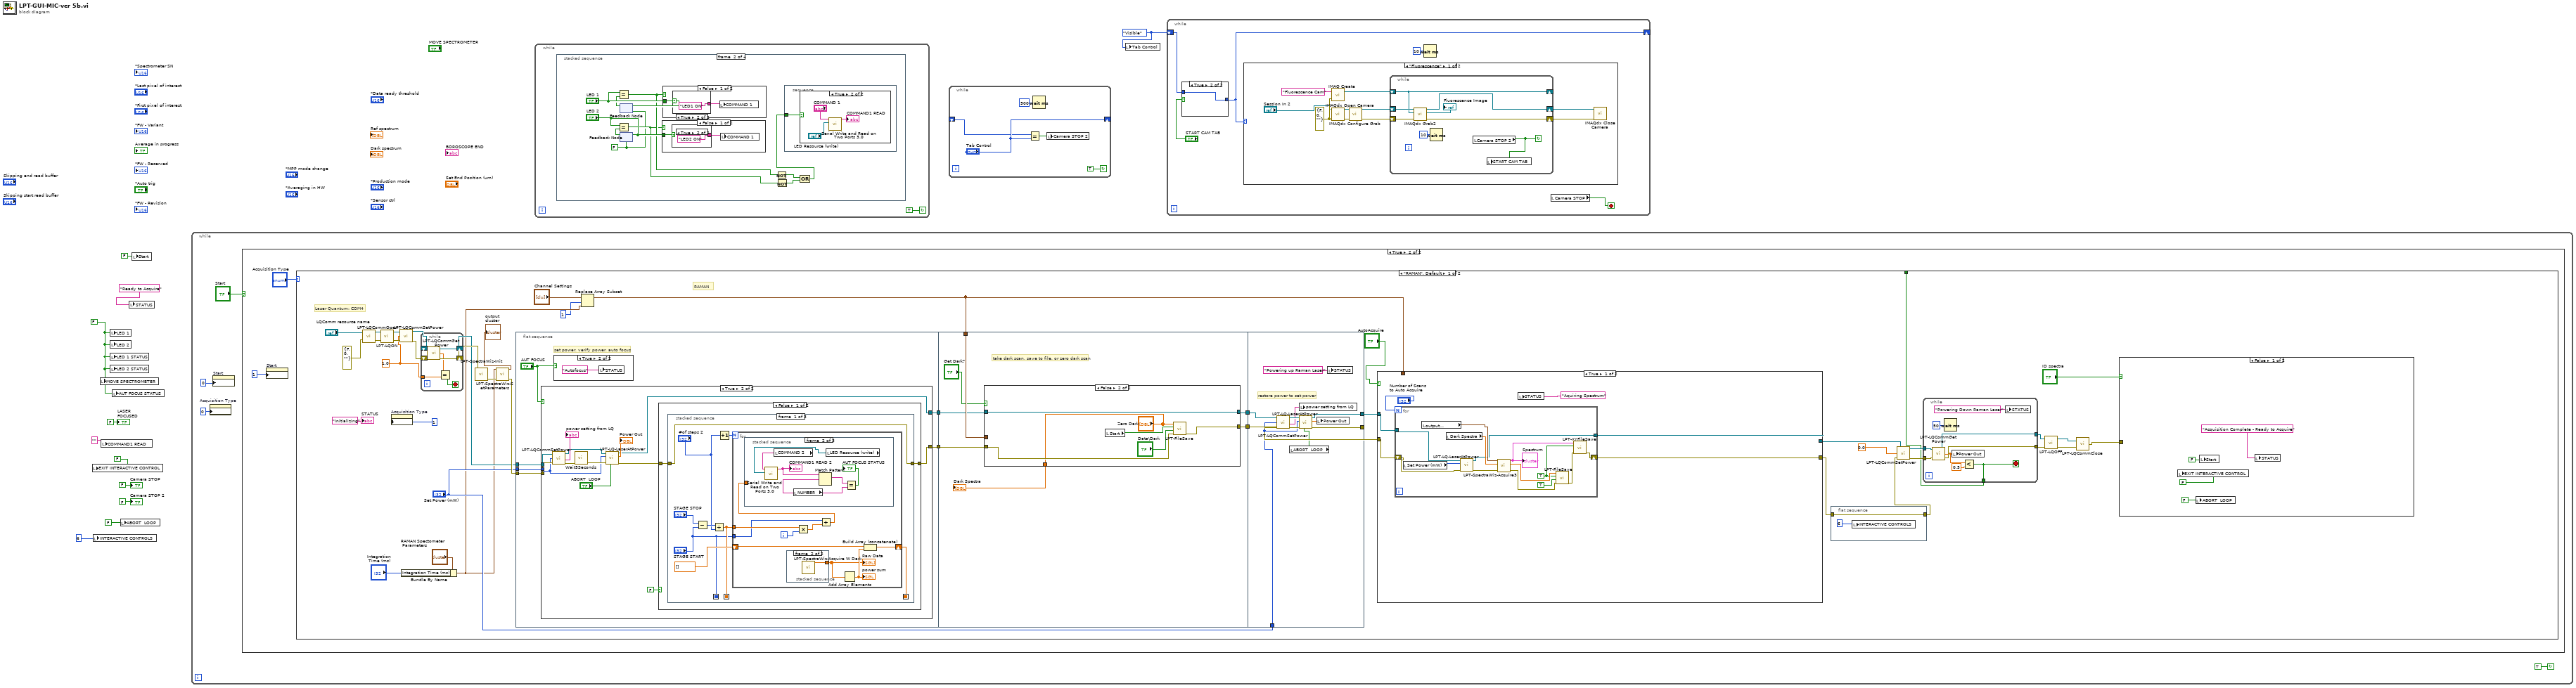
[diagram p0: block diagram]
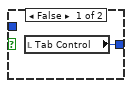
[diagram p2: hidden frame]
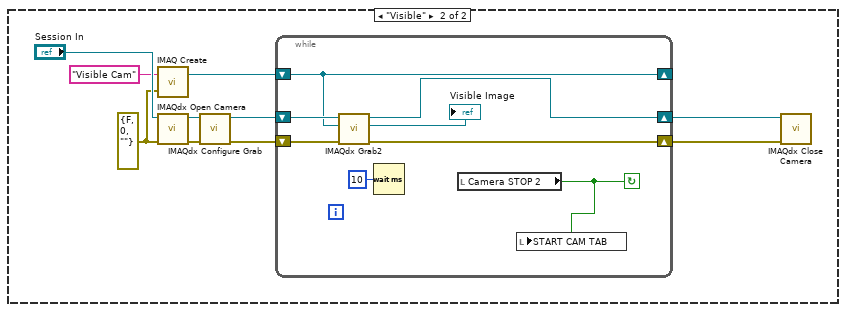
[diagram p3: hidden frame]
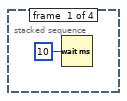
[diagram p4: hidden frame]
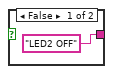
[diagram p6: hidden frame]
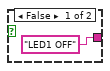
[diagram p8: hidden frame]
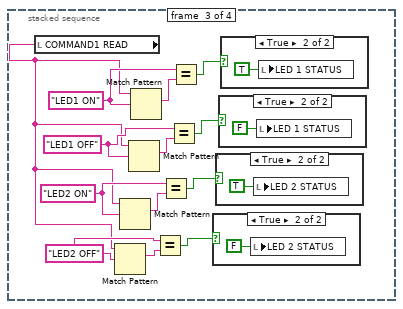
[diagram p10: hidden frame]
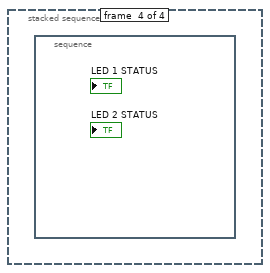
[diagram p15: hidden frame]
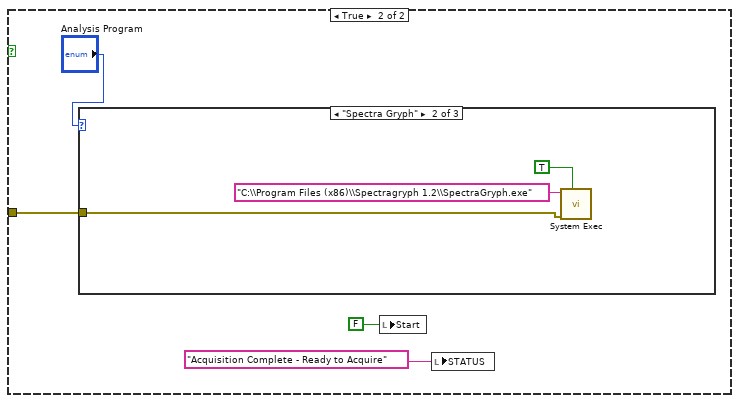
[diagram p17: hidden frame]
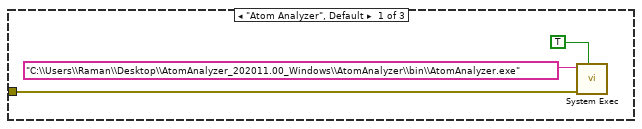
[diagram p18: hidden frame]
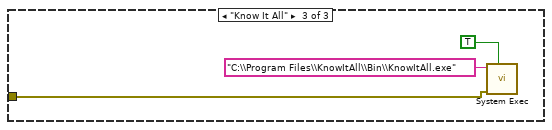
[diagram p19: hidden frame]
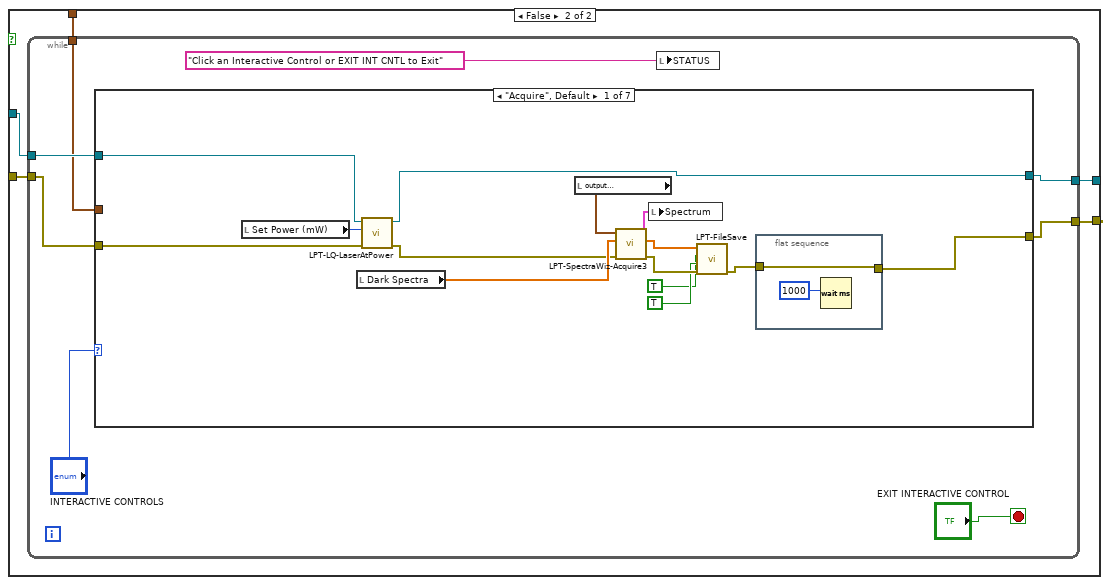
[diagram p20: hidden frame]
diagram:
  w1 = enum32{"Visible", "Fluorescence"}."Visible" ("Tab Control")
  w4 = FALSE
  n1 = local write "EXIT INTERACTIVE CONTROL"(FALSE) -> ()
  n2 = local write "INTERACTIVE CONTROLS"(6) -> ()
  n3 = local write "MOVE SPECTROMETER"(w4) -> ()
  n4 = local write "COMMAND1 READ"("" ("COMMAND1 READ")) -> ()
  n5 = local write "LED 1"(w4) -> ()
  n6 = local write "LED 2"(w4) -> ()
  n7 = local write "LED 1 STATUS"(w4) -> ()
  n8 = local write "LED 2 STATUS"(w4) -> ()
  n9 = local write "AUT FOCUS STATUS"(w4) -> ()
  n10 = local write "ABORT  LOOP"(FALSE) -> ()
  n11 = local write "STATUS"("Ready to Acquire") -> ()
  n12 = local write "Start"(FALSE) -> ()
  n13 = while {
    stop <- TRUE continue-if-true
    n14 = property on="Acquisition Type" class="RadioBtnsControl (strict)"("DisabledEnum"=0) -> ()  [unwired: 2 in, 2 out]
    n15 = property on="Start" class="Bool (strict)"("DisabledEnum"=0) -> ()  [unwired: 2 in, 2 out]
    n16 = case shown="True" "Start" {
      frame False {
      }
      frame True {
        n17 = property on="Start" class="Bool (strict)"("DisabledEnum"=1) -> ()  [unwired: 2 in, 2 out]
        n18 = case shown="\"RAMAN\", Default" "Acquisition Type" {
          tunnel: [w37 w353] -> _
          frame "RAMAN", Default {
            w32 = 1.0 ("Set Power (mW)")
            # "RAMAN"
            # "Laser Quantum: COM4"
            n19 = call "LPT-LQCommOpen.vi"("error in"=errorcluster {"status"=FALSE, "code"=0, "source"=""}, "LQComm resource name"="LQComm resource name") -> ("error out"=w54:errorcluster, "LQComm Resource out"=w55:refnum<visa-resource-name>)
            n20 = call "LPT-LQON.vi"("error in"=w54, "LQComm Resource In"=w55) -> ("error out"=w36:errorcluster, "LQComm Resource Out"=w35:refnum<visa-resource-name>)  [unwired: 1 in, 1 out]
            n21 = property on="Acquisition Type" class="RadioBtnsControl (strict)"("DisabledEnum"=1) -> ()  [unwired: 2 in, 2 out]
            n22 = call "LPT-LQCommSetPower.vi"("LQComm Resource In"=w35, "Set Power (mW)"=w32, "error in"=w36) -> ("LQComm Resource Out"=w34:refnum<visa-resource-name>, "error out"=w33:errorcluster)  [unwired: 2 out]
            n23 = Bundle By Name(cluster="RAMAN Spectometer\n Parameters", "Integration Time (ms)"="Integration\n Time (ms)") -> (w27:T6)
            n24 = while {
              shift-right: [w67] -> w30
              shift-left: w34 -> [w69]
              shift-right: [w68] -> w31
              shift-left: w33 -> [w66]
              tunnel: w32 -> [w64]
              stop <- w63 stop-if-true
              n25 = call "LPT-LQCommGetPower.vi"("error in"=w66, "LQComm Resource In"=w69) -> ("error out"=w68:errorcluster, "NumericValue"=w65:dbl, "LQComm Resource Out"=w67:refnum<visa-resource-name>)  [unwired: 1 in]
              n26 = Equal?(x=w65, y=w64) -> (x = y?=w63:bool)
            }
            n27 = call "LPT-SpectraWiz-Init.vi"("error in (no error)"=w31) -> ("error out"=w47:errorcluster)  [unwired: 10 in]
            n28 = call "LPT-SpectraWiz-SetParameters.vi"("error in"=w47, "input cluster"=w27) -> ("error out"=w46:errorcluster, "output cluster"=→"output\ncluster":T5)  [unwired: 8 in]
            n29 = flat-sequence {
              tunnel: w46 -> [w227]
              tunnel: "Set Power (mW)" -> [w228]
              tunnel: [w226] -> w60
              tunnel: [w225] -> w59
              tunnel: w30 -> [w224]
              tunnel: w18 -> [w306]
              tunnel: [w305] -> w58
              tunnel: w60 -> [w303]
              tunnel: w59 -> [w301]
              tunnel: [w302] -> w57
              tunnel: "Set Power (mW)" -> [w333]
              tunnel: w58 -> [w336]
              tunnel: [w332] -> w44
              tunnel: w57 -> [w331]
              tunnel: [w329] -> w43
              frame #0 {
                # "set power, verify power, auto focus"
                n30 = case shown="True" "AUT FOCUS" {
                  tunnel: w228 -> [_ w238]
                  tunnel: w227 -> [w231 w243]
                  tunnel: [w231 w234] -> w226
                  tunnel: [w230 w232] -> w225
                  tunnel: w224 -> [w230 w239]
                  frame False {
                  }
                  frame True {
                    n31 = call "LPT-LQCommSetPower.vi"("LQComm Resource In"=w239, "Set Power (mW)"=w238, "error in"=w243) -> ("LQComm Resource Out"=w242:refnum<visa-resource-name>, "decimal integer string"=→"power setting from LQ":string, "error out"=w241:errorcluster)  [unwired: 1 out]
                    n32 = call "Wait5Seconds.vi"("error in"=w241) -> ("error out"=w240:errorcluster)  [unwired: 10 in]
                    n33 = call "LPT-LQ-LaserAtPower.vi"("Abort Loop"="ABORT  LOOP", "error in"=w240, "Set Power (mW)"=w238, "LQComm Resource In"=w242) -> ("error out"=w235:errorcluster, "Power Out"=→"Power Out":dbl, "LQComm Resource Out"=w232:refnum<visa-resource-name>)  [unwired: 4 in, 1 out]
                    n34 = case shown="False" FALSE {
                      tunnel: w235 -> [w245 w295]
                      tunnel: [w246 w290] -> w234
                      frame False {
                        n35 = stacked-sequence {
                          seq-local: [w249 _ _] -> [_ w278 _]
                          seq-local: [w248 _ _] -> [_ w281 _]
                          seq-local: ["STAGE START" _ _] -> [_ w282 _]
                          tunnel: [w251 _ _] -> w246
                          tunnel: w245 -> [w251 _ _]
                          frame #0 {
                            n36 = Subtract(x="STAGE STOP", y="STAGE START") -> (x-y=w253:i32)
                            n37 = Divide(x=w253, y="#of steps 2") -> (x/y=w248:dbl)
                            n38 = Increment(x="#of steps 2") -> (x+1=w254:i32)
                            n39 = for {
                              N: w254 -> [_]
                              tunnel: w248 -> [w264]
                              tunnel: "STAGE START" -> [w260]
                              shift-right: [w256] -> w249
                              shift-left: sgl[] [] -> [w257]
                              i -> [w263]
                              n40 = stacked-sequence {
                                tunnel: [_ w266] -> w258
                                frame #0 {
                                n41 = Wait (ms)(milliseconds to wait=u32 1000) -> ()  [unwired: 1 out]
                                }
                                frame #1 {
                                n42 = call "LPT-SpectraWiz-Acquire W Dark.vi"() -> ("Buffer"=w266:sgl[])  [unwired: 10 in, 1 out]
                                }
                              }
                              "Raw Data" <- w258
                              n43 = Multiply(x=w264, y=w263) -> (x*y=w262:dbl)
                              n44 = Add(x=w260, y=w262) -> (x+y=w261:dbl)
                              n45 = stacked-sequence {
                                tunnel: w261 -> [w269 _ _]
                                frame #0 {
                                n46 = Number To Decimal String(number=w269) -> (decimal integer string=w268:string)  [unwired: 1 in]
                                "NUMBER" <- w268
                                n47 = Concatenate Strings("MOV ", w268) -> (→"COMMAND 2":string)
                                "Position (um)" <- w269
                                }
                                frame #1 {
                                n48 = local read "COMMAND 2"() -> (w276:string)
                                n49 = local read "NUMBER"() -> (w274:string)
                                n50 = local read "LED Resource (write)"() -> (w271:refnum<visa-resource-name>)
                                n51 = call "Serial Write and Read on Two Ports 3.0.vi"("VISA Resource (write)"=w271, "Write String"=w276) -> ("Read String"=w275:string)  [unwired: 9 in]
                                "COMMAND1 READ 2" <- w275
                                n52 = Match Pattern(string=w275, regular expression=w274) -> (match substring=w273:string)  [unwired: 1 in, 3 out]
                                n53 = Equal?(x=w273, y=w274) -> (x = y?=→"AUT FOCUS STATUS":bool)
                                }
                                frame #2 {
                                n54 = Wait (ms)(milliseconds to wait=u32 100) -> ()  [unwired: 1 out]
                                }
                              }
                              n55 = Add Array Elements(numeric array=w258) -> (sum=w259:sgl)
                              "power sum" <- w259
                              n56 = Build Array (concatenate)(w257, w259) -> (w256:sgl[])
                            }
                          }
                          frame #1 {
                            (unwired) 10.0 ("Position (mm)")
                            (unwired) 500.0 ("MaxPosition")
                            (unwired) sgl 3651732.0 ("max value")
                            n57 = Array Max & Min(array=w278) -> (max value=w280:sgl, max index (indices)=w284:i32)  [unwired: 2 out]
                            n58 = Multiply(x=w284, y=w281) -> (x*y=w283:dbl)
                            n59 = local write "max value"(w280) -> ()
                            n60 = Add(x=w283, y=w282) -> (x+y=w279:dbl)
                            n61 = local write "MaxPosition"(w279) -> ()
                            n62 = local write "Position (um)"(w279) -> ()
                          }
                          frame #2 {
                            n63 = local read "Position (um)"() -> (w286:dbl)
                            n64 = Number To Decimal String(number=w286) -> (decimal integer string=w287:string)  [unwired: 1 in]
                            n65 = Concatenate Strings("MOV ", w287) -> (w285:string)
                            n66 = call "Serial Write and Read on Two Ports 3.0.vi"("Write String"=w285) -> ()  [unwired: 10 in, 1 out]
                          }
                        }
                      }
                      frame True {
                        n67 = call "LPT-Firgelli_AutoFocus.vi"("error in (no error)"=w295, "STOP"="STAGE STOP A", "START"="STAGE START A", "#of steps"="#of steps A") -> ("error out"=w291:errorcluster, "MaxPosition"=→"MaxPosition":dbl, "max value"=→"max value":sgl, "Position (mm)"=→"Position (mm)":dbl)  [unwired: 3 in, 1 out]
                        n68 = in-place {
                          in-place-border: w291 -> [w299]
                          in-place-border: [w299] -> w290
                          n69 = local write "LASER \nFOCUSED"(TRUE ("Laser \nFocused")) -> ()
                        }
                      }
                    }
                  }
                }
                n70 = case shown="True" "AUT FOCUS" {
                  frame False {
                  }
                  frame True {
                    n71 = local write "STATUS"("Autofocus") -> ()
                  }
                }
              }
              frame #1 {
                # "take dark scan, save to file, or zero dark scan"
                n72 = case shown="False" "Get Dark?" {
                  tunnel: w306 -> [w321 _]
                  tunnel: [w317 w324] -> w305
                  tunnel: [w308 "Zero Dark"] -> w304
                  tunnel: w303 -> [w310 w325]
                  tunnel: w301 -> [w309 w327]
                  tunnel: [w309 w327] -> w302
                  frame True {
                    n73 = call "LPT-SpectraWiz-GetDark.vi"("error in"=w310, "Channel Settings"=w321, "LQComm Resource In"=w309) -> ("error out"=w318:errorcluster, "Dark Spectra"=w308:sgl[])  [unwired: 7 in]
                    n74 = local write "STATUS"("Getting Dark Spectrum") -> ()
                    n75 = Format Date/Time String(time format string (%c)="%y%m%d%H%M%S") -> (date/time string=w314:string)  [unwired: 2 in]
                    n76 = Concatenate Strings(w314, "Raman" ("string"), "Dark" ("string")) -> (w316:string)
                    n77 = Build Path(base path=path "C:/Program Files (x86)/National Instruments/LabVIEW 2019/instr.lib/LPT/DataRaman", name or relative path=w316) -> (appended path=w320:path)
                    n78 = call-poly <vilib>:"Write Delimited Spreadsheet.vi"("file path (dialog if empty)"=w320, "1D data"=w308, "error in (no error)"=w318, "transpose? (no:F)"=TRUE) -> ("error out"=w317:errorcluster)  [unwired: 10 in, 1 out]
                  }
                  frame False {
                    n79 = local read "Start"() -> (w322:bool)
                    n80 = call "LPT-FileSave.vi"("error in (no error)"=w325, "Data\\Dark"="Data\\Dark", "Raman\\LIBS"=w322, "Array"="Zero Dark") -> ("error out"=w324:errorcluster)  [unwired: 7 in]
                  }
                }
                "Dark Spectra" <- w304
              }
              frame #2 {
                # "restore power to set power"
                n81 = call "LPT-LQCommSetPower.vi"("LQComm Resource In"=w331, "Set Power (mW)"=w333, "error in"=w336) -> ("LQComm Resource Out"=w337:refnum<visa-resource-name>, "decimal integer string"=w334:string, "error out"=w338:errorcluster)  [unwired: 1 out]
                n82 = local read "ABORT  LOOP"() -> (w330:bool)
                n83 = local write "power setting from LQ"(w334) -> ()
                n84 = call "LPT-LQ-LaserAtPower.vi"("Abort Loop"=w330, "error in"=w338, "Set Power (mW)"=w333, "LQComm Resource In"=w337) -> ("error out"=w332:errorcluster, "Power Out"=w335:dbl, "LQComm Resource Out"=w329:refnum<visa-resource-name>)  [unwired: 4 in, 1 out]
                n85 = local write "Power Out"(w335) -> ()
                n86 = local write "STATUS"("Powering up Raman Laser" ("STATUS")) -> ()
              }
            }
            n87 = Replace Array Subset(array="Channel Settings", new element=w27, index=u32 1 ("Channel\n(1-based)")) -> (w18:T4)
            n88 = case shown="True" "AutoAcquire" {
              tunnel: [w92 w111] -> w20
              tunnel: w44 -> [w87 w110]
              tunnel: w43 -> [w91 w109]
              tunnel: [w88 w108] -> w38
              tunnel: w18 -> [_ w107]
              frame True {
                n89 = for {
                  N: "Number of Scans \nto Auto Acquire" -> [_]
                  tunnel: w91 -> [w105]
                  shift-right: [w94] -> w92
                  shift-left: w87 -> [w106]
                  tunnel: [w93] -> w88
                  w96 = TRUE ("Raman\\LIBS")
                  n90 = local read "Set Power (mW)"() -> (w103:i32)
                  n91 = local read "output\ncluster"() -> (w98:T5)
                  n92 = local read "Dark Spectra"() -> (w102:dbl[])
                  n93 = call "LPT-LQ-LaserAtPower.vi"("error in"=w106, "Set Power (mW)"=w103, "LQComm Resource In"=w105) -> ("error out"=w104:errorcluster, "LQComm Resource Out"=w93:refnum<visa-resource-name>)  [unwired: 5 in, 2 out]
                  n94 = call "LPT-SpectraWiz-Acquire3.vi"("error in"=w104, "Dark Array"=w102, "input cluster"=w98) -> ("error out"=w100:errorcluster, "Raw Data"=w101:sgl[], "Spectrum"=w97:cluster{dbl[], "Dark Array":dbl[]})  [unwired: 5 in, 1 out]
                  "Spectrum" <- w97
                  n95 = call "LPT-FileSave.vi"("error in (no error)"=w100, "Data\\Dark"=TRUE ("Data\\Dark"), "Raman\\LIBS"=w96, "Array"=w101) -> ("error out"=w95:errorcluster)  [unwired: 7 in]
                  n96 = call "LPT-XYFileSave.vi"("error in (no error)"=w95, "Raman\\LIBS"=w96, "Spectrum"=w97) -> ("error out"=w94:errorcluster)  [unwired: 8 in]
                }
                n97 = local write "STATUS"("Aquiring Spectrum" ("STATUS")) -> ()
              }
              frame False {
                n98 = while {
                  tunnel: [w114] -> w111
                  tunnel: w110 -> [w116]
                  tunnel: w109 -> [w115]
                  tunnel: [w113] -> w108
                  tunnel: w107 -> [w112]
                  stop <- "EXIT INTERACTIVE CONTROL" stop-if-true
                  n99 = case shown="\"Acquire\", Default" "INTERACTIVE CONTROLS" {
                    tunnel: w116 -> [w123 w141 w163 w175 w194 w202 w219]
                    tunnel: w115 -> [w122 w140 w162 w176 w193 w201 w220]
                    tunnel: [w121 w136 w159 w187 w191 w199 w218] -> w114
                    tunnel: [w120 w140 w161 w176 w193 w201 w220] -> w113
                    tunnel: w112 -> [_ _ _ w173 _ _ _]
                    frame "Acquire", Default {
                      n100 = local read "Set Power (mW)"() -> (w127:i32)
                      n101 = local read "Dark Spectra"() -> (w128:dbl[])
                      n102 = call "LPT-LQ-LaserAtPower.vi"("error in"=w123, "Set Power (mW)"=w127, "LQComm Resource In"=w122) -> ("error out"=w126:errorcluster, "LQComm Resource Out"=w120:refnum<visa-resource-name>)  [unwired: 5 in, 2 out]
                      n103 = local read "output\ncluster"() -> (w130:T5)
                      n104 = call "LPT-SpectraWiz-Acquire3.vi"("error in"=w126, "Dark Array"=w128, "input cluster"=w130) -> ("error out"=w129:errorcluster, "Raw Data"=w132:sgl[], "Spectrum"=w131:cluster{dbl[], "Dark Array":dbl[]})  [unwired: 5 in, 1 out]
                      n105 = local write "Spectrum"(w131) -> ()
                      n106 = call "LPT-FileSave.vi"("error in (no error)"=w129, "Data\\Dark"=TRUE ("Data\\Dark"), "Raman\\LIBS"=TRUE ("Raman\\LIBS"), "Array"=w132) -> ("error out"=w133:errorcluster)  [unwired: 7 in]
                      n107 = flat-sequence {
                        tunnel: w133 -> [w134]
                        tunnel: [w134] -> w121
                        frame #0 {
                          n108 = Wait (ms)(milliseconds to wait=1000) -> ()  [unwired: 1 out]
                        }
                      }
                    }
                    frame "ReFocus" {
                      n109 = local read "Set End Position (um)"() -> (w146:dbl)
                      n110 = Less?(x=w146, y=2) -> (x < y?=w145:bool)
                      n111 = case shown="False" w145 {
                        tunnel: w146 -> [w155 _]
                        tunnel: [w153 1] -> w147
                        tunnel: [w152 3] -> w148
                        frame False {
                          n112 = Subtract(x=w155, y=1) -> (x-y=w153:dbl)
                          n113 = Add(x=w153, y=2) -> (x+y=w152:dbl)
                        }
                        frame True {
                        }
                      }
                      n114 = call "LPT-Firgelli_AutoFocus.vi"("error in (no error)"=w141, "STOP"=w148, "START"=w147, "#of steps"=10) -> ("error out"=w137:errorcluster, "MaxPosition"=w144:dbl, "max value"=w143:sgl, "Position (mm)"=w142:dbl)  [unwired: 3 in, 1 out]
                      n115 = local write "Set End Position (um)"(w142) -> ()
                      n116 = local write "max value"(w143) -> ()
                      n117 = local write "MaxPosition"(w144) -> ()
                      n118 = flat-sequence {
                        tunnel: w137 -> [w151]
                        tunnel: [w151] -> w136
                        frame #0 {
                          n119 = local write "INTERACTIVE CONTROLS"(6) -> ()
                          n120 = Wait (ms)(milliseconds to wait=1000) -> ()  [unwired: 1 out]
                        }
                      }
                    }
                    frame "ReSet Power" {
                      n121 = local read "Set Power (mW)"() -> (w167:i32)
                      n122 = local read "ABORT  LOOP"() -> (w164:bool)
                      n123 = call "LPT-LQCommSetPower.vi"("LQComm Resource In"=w162, "Set Power (mW)"=w167, "error in"=w163) -> ("LQComm Resource Out"=w168:refnum<visa-resource-name>, "decimal integer string"=w166:string, "error out"=w169:errorcluster)  [unwired: 1 out]
                      n124 = local write "power setting from LQ"(w166) -> ()
                      n125 = call "LPT-LQ-LaserAtPower.vi"("Abort Loop"=w164, "error in"=w169, "Set Power (mW)"=w167, "LQComm Resource In"=w168) -> ("error out"=w160:errorcluster, "Power Out"=w165:dbl, "LQComm Resource Out"=w161:refnum<visa-resource-name>)  [unwired: 4 in, 1 out]
                      n126 = local write "Power Out"(w165) -> ()
                      n127 = flat-sequence {
                        tunnel: [w172] -> w159
                        tunnel: w160 -> [w172]
                        frame #0 {
                          n128 = local write "INTERACTIVE CONTROLS"(6) -> ()
                          n129 = Wait (ms)(milliseconds to wait=1000) -> ()  [unwired: 1 out]
                        }
                      }
                    }
                    frame "New Dark" {
                      n130 = call "LPT-SpectraWiz-GetDark.vi"("error in"=w175, "Channel Settings"=w173, "LQComm Resource In"=w176) -> ("error out"=w184:errorcluster, "Dark Spectra"=w177:sgl[])  [unwired: 7 in]
                      n131 = local write "Dark spectrum"(w177) -> ()
                      n132 = Format Date/Time String(time format string (%c)="%y%m%d%H%M%S") -> (date/time string=w181:string)  [unwired: 2 in]
                      n133 = Concatenate Strings(w181, "Raman" ("string"), "Dark" ("string")) -> (w183:string)
                      n134 = Build Path(base path=path "C:/Program Files (x86)/National Instruments/LabVIEW 2019/instr.lib/LPT/DataRaman", name or relative path=w183) -> (appended path=w186:path)
                      n135 = call-poly <vilib>:"Write Delimited Spreadsheet.vi"("file path (dialog if empty)"=w186, "1D data"=w177, "error in (no error)"=w184, "transpose? (no:F)"=TRUE) -> ("error out"=w174:errorcluster)  [unwired: 10 in, 1 out]
                      n136 = flat-sequence {
                        tunnel: w174 -> [w190]
                        tunnel: [w190] -> w187
                        frame #0 {
                          n137 = local write "INTERACTIVE CONTROLS"(6) -> ()
                          n138 = Wait (ms)(milliseconds to wait=1000) -> ()  [unwired: 1 out]
                        }
                      }
                    }
                    frame "Parameter Reset" {
                      n139 = local read "output\ncluster"() -> (w195:T5)
                      n140 = call "LPT-SpectraWiz-SetParameters.vi"("error in"=w194, "input cluster"=w195) -> ("error out"=w192:errorcluster)  [unwired: 8 in, 1 out]
                      n141 = flat-sequence {
                        tunnel: w192 -> [w198]
                        tunnel: [w198] -> w191
                        frame #0 {
                          n142 = local write "INTERACTIVE CONTROLS"(6) -> ()
                          n143 = Wait (ms)(milliseconds to wait=1000) -> ()  [unwired: 1 out]
                        }
                      }
                    }
                    frame "Material ID" {
                      n144 = local read "Analysis Program"() -> (w203:T3)
                      n145 = case shown="\"Atom Analyzer\", Default" w203 {
                        tunnel: w202 -> [w207 w211 w215]
                        tunnel: [w206 w210 w214] -> w200
                        frame "Atom Analyzer", Default {
                          n146 = call <vilib>:"System Exec.vi"("wait until completion? (T)"=TRUE, "error in (no error)"=w207, "command line"="C:\\Users\\Raman\\Desktop\\AtomAnalyzer_202011.00_Windows\\AtomAnalyzer\\bin\\AtomAnalyzer.exe") -> ("error out"=w206:errorcluster)  [unwired: 5 in, 3 out]
                        }
                        frame "Spectra Gryph" {
                          n147 = call <vilib>:"System Exec.vi"("wait until completion? (T)"=TRUE, "error in (no error)"=w211, "command line"="C:\\Program Files (x86)\\Spectragryph 1.2\\SpectraGryph.exe" ("standard input")) -> ("error out"=w210:errorcluster)  [unwired: 5 in, 3 out]
                        }
                        frame "Know It All" {
                          n148 = call <vilib>:"System Exec.vi"("wait until completion? (T)"=TRUE, "error in (no error)"=w215, "command line"="C:\\Program Files\\KnowItAll\\Bin\\KnowItAll.exe") -> ("error out"=w214:errorcluster)  [unwired: 5 in, 3 out]
                        }
                      }
                      n149 = flat-sequence {
                        tunnel: w200 -> [w205]
                        tunnel: [w205] -> w199
                        frame #0 {
                          n150 = local write "INTERACTIVE CONTROLS"(6) -> ()
                        }
                      }
                    }
                    frame "Do Nothing" {
                      n151 = flat-sequence {
                        tunnel: w219 -> [w222]
                        tunnel: [w222] -> w218
                        frame #0 {
                          n152 = Wait (ms)(milliseconds to wait=500) -> ()  [unwired: 1 out]
                        }
                      }
                    }
                  }
                  n153 = local write "STATUS"("Click an Interactive Control or EXIT INT CNTL to Exit" ("STATUS")) -> ()
                }
              }
            }
            n154 = flat-sequence {
              tunnel: w20 -> [w61]
              tunnel: [w61] -> w19
              frame #0 {
                n155 = local write "INTERACTIVE CONTROLS"(6) -> ()
              }
            }
            n156 = call "LPT-LQCommSetPower.vi"("LQComm Resource In"=w38, "Set Power (mW)"=0.0, "error in"=w19) -> ("LQComm Resource Out"=w52:refnum<visa-resource-name>, "error out"=w51:errorcluster)  [unwired: 2 out]
            n157 = while {
              tunnel: w52 -> [w347]
              tunnel: w51 -> [w346]
              tunnel: [w343] -> w50
              tunnel: [w342] -> w49
              tunnel: [w339] -> w37
              stop <- w339 stop-if-true
              n158 = call "LPT-LQCommGetPower.vi"("error in"=w346, "LQComm Resource In"=w347) -> ("error out"=w342:errorcluster, "NumericValue"=w341:dbl, "LQComm Resource Out"=w343:refnum<visa-resource-name>)  [unwired: 1 in]
              n159 = Wait (ms)(milliseconds to wait=u32 50) -> ()  [unwired: 1 out]
              n160 = local write "Power Out"(w341) -> ()
              n161 = Less?(x=w341, y=0.5) -> (x < y?=w339:bool)
              n162 = local write "STATUS"("Powering Down Raman Laser" ("STATUS")) -> ()
            }
            n163 = call "LPT-LQOFF.vi"("error in"=w49, "LQComm Resource In"=w50) -> ("error out"=w40:errorcluster, "LQComm Resource Out"=w53:refnum<visa-resource-name>)  [unwired: 1 in, 1 out]
            n164 = call "LPT-LQCommClose.vi"("error in (no error)"=w40, "LQ Resource In"=w53) -> ("error out"=w21:errorcluster)
            n165 = case shown="False" "ID spectra" {
              tunnel: w21 -> [_ w75]
              frame False {
                n166 = local write "EXIT INTERACTIVE CONTROL"(FALSE) -> ()
                n167 = local write "ABORT  LOOP"(FALSE) -> ()
                n168 = local write "Start"(FALSE) -> ()
                n169 = local write "STATUS"("Acquisition Complete - Ready to Acquire") -> ()
              }
              frame True {
                n170 = case shown="\"Spectra Gryph\"" "Analysis Program" {
                  tunnel: w75 -> [w78 w81 w84]
                  frame "Atom Analyzer", Default {
                    n171 = call <vilib>:"System Exec.vi"("wait until completion? (T)"=TRUE, "error in (no error)"=w78, "command line"="C:\\Users\\Raman\\Desktop\\AtomAnalyzer_202011.00_Windows\\AtomAnalyzer\\bin\\AtomAnalyzer.exe" ("standard input")) -> ()  [unwired: 5 in, 4 out]
                  }
                  frame "Spectra Gryph" {
                    n172 = call <vilib>:"System Exec.vi"("wait until completion? (T)"=TRUE, "error in (no error)"=w81, "command line"="C:\\Program Files (x86)\\Spectragryph 1.2\\SpectraGryph.exe" ("standard input")) -> ()  [unwired: 5 in, 4 out]
                  }
                  frame "Know It All" {
                    n173 = call <vilib>:"System Exec.vi"("wait until completion? (T)"=TRUE, "error in (no error)"=w84, "command line"="C:\\Program Files\\KnowItAll\\Bin\\KnowItAll.exe" ("standard input")) -> ()  [unwired: 5 in, 4 out]
                  }
                }
                n174 = local write "Start"(FALSE) -> ()
                n175 = local write "STATUS"("Acquisition Complete - Ready to Acquire") -> ()
              }
            }
            "STATUS" <- "Initializing"
          }
          frame "LIBS" {
            # "Turn off\nfunc. gen"
            # "set power level of LIBS by adjusting the pulse rate until a suitable signal level in the spectrometer is obtained, it is assumed that Raman will be performed first, getting the lens approximately into focus position."
            # "LIBS"
            n176 = flat-sequence {
              tunnel: [w508] -> w361
              tunnel: [w507] -> w360
              tunnel: [w506] -> w359
              tunnel: errorcluster {"status"=FALSE, "code"=0, "source"=""} ("error in") -> [w505]
              tunnel: w361 -> [w549]
              tunnel: w360 -> [w548]
              tunnel: w359 -> [w547]
              tunnel: [w527] -> w355
              tunnel: [w912] -> w356
              tunnel: w355 -> [w910]
              tunnel: w356 -> [w936]
              tunnel: [w933] -> w362
              frame #0 {
                w521 = FALSE  # Write/Read (Get=true)
                # "Make sure \nfunction gen\nis off"
                # "Starting with\n slow speed"
                n177 = call "labview dds-3x25 LPT.vi"("error in (no error)"=w505, "Frequency"=0) -> ("error out"=w504:errorcluster)  [unwired: 1 in]
                n178 = call "Init.vi"("error in (no error)"=w504, "SPI frequency"=u32 4800000) -> ("error out"=w513:errorcluster, "port out"=w514:u8, "handle"=w515:u16)  [unwired: 6 in, 1 out]
                n179 = call "Spi_Config.vi"("error in (no error)"=w513, "port"=w514, "Handle"=w515) -> ("error out"=w512:errorcluster, "port out"=w510:u8, "handle"=w511:u16)  [unwired: 6 in]
                n180 = call "Set or Get SPI Register_3.vi"("Write data (16 bit)"=u16 16, "Write/Read (Get=true)"=w521, "error in (no error)"=w512, "Register name"=Register_name."Sensor ctrl", "port"=w510, "Handle"=w511) -> ("error out"=w518:errorcluster, "port out"=w517:u8, "handle out"=w516:u16)  [unwired: 2 in, 1 out]
                n181 = local write "STATUS"("INITIALIZING LIBS") -> ()
                n182 = stacked-sequence {
                  tunnel: w518 -> [w524]
                  tunnel: w517 -> [w526]
                  tunnel: w516 -> [w525]
                  tunnel: [w526] -> w508
                  tunnel: [w525] -> w507
                  tunnel: [w524] -> w506
                  frame #0 {
                    n183 = Wait (ms)(milliseconds to wait=u32 100) -> ()  [unwired: 1 out]
                  }
                }
              }
              frame #1 {
                w550 = Register_name."Serial number"  # Register name
                n184 = while {
                  tunnel: w548 -> [w610]
                  tunnel: w549 -> [w609]
                  tunnel: w547 -> [w608]
                  shift-right: [w607] -> _
                  shift-left: w550 -> [w606]
                  tunnel: [w604] -> w536
                  tunnel: [w603] -> w537
                  tunnel: [w602] -> w538
                  tunnel: [w601] -> w532
                  tunnel: [w600] -> w534
                  tunnel: [w599] -> w533
                  stop <- w601 stop-if-true
                  n185 = case shown="\"SPECTROMETER SN\"" w606 {
                    selector: w606 -> [w613 w621 w630 w656 w667 w682 w693 w701 w720 w731 w742 w753 w764 w775 w786 w797 w808 w819 w830 w846 w857 w868 w879 w890 w902]
                    tunnel: w610 -> [w612 w625 w636 w662 w673 w688 w699 w707 w726 w737 w748 w759 w770 w781 w792 w803 w814 w825 w836 w852 w863 w874 w885 w896 w907]
                    tunnel: w609 -> [w611 w624 w635 w661 w672 w687 w698 w706 w725 w736 w747 w758 w769 w780 w791 w802 w813 w824 w835 w851 w862 w873 w884 w895 w906]
                    tunnel: w608 -> [w615 w623 w634 w660 w671 w686 w697 w705 w724 w735 w746 w757 w768 w779 w790 w801 w812 w823 w834 w850 w861 w872 w883 w894 w905]
                    tunnel: [w613 w622 w633 w657 w668 w683 w694 w713 w721 w732 w743 w754 w765 w776 w787 w798 w809 w820 w831 w847 w858 w869 w880 w891 Register_name."Serial number" ("Register name")] -> w607
                    tunnel: [FALSE FALSE FALSE FALSE FALSE FALSE FALSE FALSE FALSE FALSE FALSE FALSE FALSE FALSE FALSE FALSE FALSE FALSE FALSE FALSE FALSE FALSE FALSE FALSE TRUE] -> w605
                    tunnel: [w615 w620 w632 w658 w669 w684 w695 w714 w722 w733 w744 w755 w766 w777 w788 w799 w810 w821 w832 w848 w859 w870 w881 w892 w903] -> w602
                    tunnel: [w612 w617 w628 w655 w665 w681 w692 w712 w719 w730 w740 w751 w763 w774 w785 w796 w807 w818 w829 w845 w856 w867 w878 w889 w901] -> w604
                    tunnel: [w611 w616 w627 w654 w664 w680 w691 w711 w718 w729 w739 w750 w762 w773 w784 w795 w806 w817 w828 w844 w855 w866 w877 w888 w900] -> w603
                    frame Default {
                    }
                    frame "Serial number" {
                      w622 = Register_name."HW version"  # Register name
                      w626 = TRUE  # Write/Read  (Get=true)
                      n186 = call "Set or Get SPI Register_3.vi"("Write/Read (Get=true)"=w626, "error in (no error)"=w623, "Register name"=w621, "port"=w624, "Handle"=w625) -> ("error out"=w620:errorcluster, "Read Data (16 bit)"=→"*PCB SN":u16, "port out"=w616:u8, "handle out"=w617:u16)  [unwired: 3 in]
                    }
                    frame "HW version" {
                      w633 = Register_name."FW version"  # Register name
                      w637 = TRUE  # Write/Read  (Get=true)
                      n187 = call "Set or Get SPI Register_3.vi"("Write/Read (Get=true)"=w637, "error in (no error)"=w634, "Register name"=w630, "port"=w635, "Handle"=w636) -> ("error out"=w632:errorcluster, "Read Data (16 bit)"=→"*HW version":u16, "port out"=w627:u8, "handle out"=w628:u16)  [unwired: 3 in]
                    }
                    frame "FW version" {
                      w657 = Register_name."Detector type"  # Register name
                      w663 = TRUE  # Write/Read  (Get=true)
                      n188 = call "Set or Get SPI Register_3.vi"("Write/Read (Get=true)"=w663, "error in (no error)"=w660, "Register name"=w656, "port"=w661, "Handle"=w662) -> ("error out"=w658:errorcluster, "Read Data (16 bit)"=w648:u16, "port out"=w654:u8, "handle out"=w655:u16)  [unwired: 3 in]
                      "*FW version" <- w648
                      n189 = Split Number(x=w648) -> (hi(x)=w653:u8, lo(x)=w650:u8)
                      n190 = local write "*FW - Revision"(w650) -> ()
                      n191 = Number To Boolean Array(number=w653) -> (Boolean array=w652:bool[])
                      n192 = Index Array(array=w652) -> (element #1=w647:bool, element #2=w646:bool, element #3=w645:bool, element #4=w644:bool, element #5=w643:bool, element #6=w640:bool, element #7=w639:bool, element #8=w638:bool)  [unwired: 8 in]
                      n193 = Build Array(w647, w646, w645, w644, w643) -> (w651:bool[])
                      n194 = Build Array(w640, w639, w638) -> (w642:bool[])
                      n195 = Boolean Array To Number(Boolean array=w651) -> (number=w649:u32)
                      n196 = Boolean Array To Number(Boolean array=w642) -> (number=w641:u32)
                      n197 = local write "*FW - Variant"(w649) -> ()
                      n198 = local write "*FW - Reserved"(w641) -> ()
                    }
                    frame "Detector type" {
                      w668 = Register_name."Pixel per image"  # Register name
                      w674 = TRUE  # Write/Read  (Get=true)
                      n199 = call "Set or Get SPI Register_3.vi"("Write/Read (Get=true)"=w674, "error in (no error)"=w671, "Register name"=w667, "port"=w672, "Handle"=w673) -> ("error out"=w669:errorcluster, "Read Data (16 bit)"=→"*Detector type":u16, "port out"=w664:u8, "handle out"=w665:u16)  [unwired: 3 in]
                    }
                    frame "Pixel per image" {
                      w683 = Register_name."Calib data chars"  # Register name
                      w689 = TRUE  # Write/Read  (Get=true)
                      n200 = call "Set or Get SPI Register_3.vi"("Write/Read (Get=true)"=w689, "error in (no error)"=w686, "Register name"=w682, "port"=w687, "Handle"=w688) -> ("error out"=w684:errorcluster, "Read Data (16 bit)"=w677:u16, "port out"=w680:u8, "handle out"=w681:u16)  [unwired: 3 in]
                      "*Pixels per image" <- w677
                      n201 = Initialize Array(0.0 ("element"), w677) -> (w676:dbl[])
                      n202 = Initialize Array(1.0 ("element"), w677) -> (w675:dbl[])
                      n203 = local write "Dark spectrum"(w676) -> ()
                      n204 = local write "Ref spectrum"(w675) -> ()
                    }
                    frame "Calib data chars" {
                      w694 = Register_name."Sensor ctrl"  # Register name
                      w700 = TRUE  # Write/Read (Get=true)
                      n205 = call "Set or Get SPI Register_3.vi"("Write/Read (Get=true)"=w700, "error in (no error)"=w697, "Register name"=w693, "port"=w698, "Handle"=w699) -> ("error out"=w695:errorcluster, "Read Data (16 bit)"=→"*Calib data chars":u16, "port out"=w691:u8, "handle out"=w692:u16)  [unwired: 3 in]
                    }
                    frame "Sensor ctrl" {
                      w709 = FALSE  # Write/Read  (Get=true)
                      w713 = Register_name."Sensor exp time LSB"  # Register name
                      w716 = TRUE  # Write/Read  (Get=true)
                      n206 = call "Set or Get SPI Register_3.vi"("Write data (16 bit)"=u16 16, "Write/Read (Get=true)"=w709, "error in (no error)"=w705, "Register name"=w701, "port"=w706, "Handle"=w707) -> ("error out"=w704:errorcluster, "port out"=w703:u8, "handle out"=w702:u16)  [unwired: 2 in, 1 out]
                      n207 = call "Set or Get SPI Register_3.vi"("Write/Read (Get=true)"=w716, "error in (no error)"=w704, "Register name"=w701, "port"=w703, "Handle"=w702) -> ("error out"=w714:errorcluster, "Read Data (16 bit)"=w710:u16, "port out"=w711:u8, "handle out"=w712:u16)  [unwired: 3 in]
                      n208 = local write "*Sensor ctrl"(w710) -> ()
                    }
                    frame "Sensor exp time LSB" {
                      w721 = Register_name."Sensor exp time MSB"  # Register name
                      w727 = TRUE  # Write/Read  (Get=true)
                      n209 = call "Set or Get SPI Register_3.vi"("Write/Read (Get=true)"=w727, "error in (no error)"=w724, "Register name"=w720, "port"=w725, "Handle"=w726) -> ("error out"=w722:errorcluster, "Read Data (16 bit)"=→"Sensor exp time LSB":u16, "port out"=w718:u8, "handle out"=w719:u16)  [unwired: 3 in]
                    }
                    frame "Sensor exp time MSB" {
                      w732 = Register_name."Temperature"  # Register name
                      w738 = TRUE  # Write/Read  (Get=true)
                      n210 = call "Set or Get SPI Register_3.vi"("Write/Read (Get=true)"=w738, "error in (no error)"=w735, "Register name"=w731, "port"=w736, "Handle"=w737) -> ("error out"=w733:errorcluster, "Read Data (16 bit)"=→"Sensor exp time MSB":u16, "port out"=w729:u8, "handle out"=w730:u16)  [unwired: 3 in]
                    }
                    frame "Temperature" {
                      w743 = Register_name."Pixel ready"  # Register name
                      w749 = TRUE  # Write/Read  (Get=true)
                      n211 = call "Set or Get SPI Register_3.vi"("Write/Read (Get=true)"=w749, "error in (no error)"=w746, "Register name"=w742, "port"=w747, "Handle"=w748) -> ("error out"=w744:errorcluster, "Read Data (16 bit)"=→"*Temperature  [counts] \n(12 bit ADC)":u16, "port out"=w739:u8, "handle out"=w740:u16)  [unwired: 3 in]
                    }
                    frame "Pixel ready" {
                      w754 = Register_name."Trigger delay LSB"  # Register name
                      w760 = TRUE  # Write/Read  (Get=true)
                      # "This indicator cannot actually \nbe used in this program"
                      n212 = call "Set or Get SPI Register_3.vi"("Write/Read (Get=true)"=w760, "error in (no error)"=w757, "Register name"=w753, "port"=w758, "Handle"=w759) -> ("error out"=w755:errorcluster, "Read Data (16 bit)"=→"Pixels ready":u16, "port out"=w750:u8, "handle out"=w751:u16)  [unwired: 3 in]
                    }
                    frame "Trigger delay LSB" {
                      w765 = Register_name."Trigger delay MSB"  # Register name
                      w771 = TRUE  # Write/Read  (Get=true)
                      n213 = call "Set or Get SPI Register_3.vi"("Write/Read (Get=true)"=w771, "error in (no error)"=w768, "Register name"=w764, "port"=w769, "Handle"=w770) -> ("error out"=w766:errorcluster, "Read Data (16 bit)"=→"Trigger delay LSB":u16, "port out"=w762:u8, "handle out"=w763:u16)  [unwired: 3 in]
                    }
                    frame "Trigger delay MSB" {
                      w776 = Register_name."ADC PGA"  # Register name
                      w782 = TRUE  # Write/Read  (Get=true)
                      n214 = call "Set or Get SPI Register_3.vi"("Write/Read (Get=true)"=w782, "error in (no error)"=w779, "Register name"=w775, "port"=w780, "Handle"=w781) -> ("error out"=w777:errorcluster, "Read Data (16 bit)"=→"Trigger delay MSB":u16, "port out"=w773:u8, "handle out"=w774:u16)  [unwired: 3 in]
                    }
                    frame "ADC PGA" {
                      w787 = Register_name."ADC offset"  # Register name
                      w793 = TRUE  # Write/Read  (Get=true)
                      n215 = call "Set or Get SPI Register_3.vi"("Write/Read (Get=true)"=w793, "error in (no error)"=w790, "Register name"=w786, "port"=w791, "Handle"=w792) -> ("error out"=w788:errorcluster, "Read Data (16 bit)"=→"*ADC gain [counts]":u16, "port out"=w784:u8, "handle out"=w785:u16)  [unwired: 3 in]
                    }
                    frame "ADC offset" {
                      w798 = Register_name."MPP mode change"  # Register name
                      w804 = TRUE  # Write/Read  (Get=true)
                      n216 = call "Set or Get SPI Register_3.vi"("Write/Read (Get=true)"=w804, "error in (no error)"=w801, "Register name"=w797, "port"=w802, "Handle"=w803) -> ("error out"=w799:errorcluster, "Read Data (16 bit)"=→"*ADC offset [counts]":u16, "port out"=w795:u8, "handle out"=w796:u16)  [unwired: 3 in]
                    }
                    frame "MPP mode change" {
                      w809 = Register_name."DATA READY THRESHOLD"  # Register name
                      w815 = TRUE  # Write/Read  (Get=true)
                      n217 = call "Set or Get SPI Register_3.vi"("Write/Read (Get=true)"=w815, "error in (no error)"=w812, "Register name"=w808, "port"=w813, "Handle"=w814) -> ("error out"=w810:errorcluster, "Read Data (16 bit)"=w805:u16, "port out"=w806:u8, "handle out"=w807:u16)  [unwired: 3 in]
                      n218 = local write "*MPP mode change"(w805) -> ()
                    }
                    frame "DATA READY THRESHOLD" {
                      w820 = Register_name."IMAGES_TO_AVERAGE"  # Register name
                      w826 = TRUE  # Write/Read  (Get=true)
                      n219 = call "Set or Get SPI Register_3.vi"("Write/Read (Get=true)"=w826, "error in (no error)"=w823, "Register name"=w819, "port"=w824, "Handle"=w825) -> ("error out"=w821:errorcluster, "Read Data (16 bit)"=w816:u16, "port out"=w817:u8, "handle out"=w818:u16)  [unwired: 3 in]
                      n220 = local write "*Data ready threshold"(w816) -> ()
                    }
                    frame "IMAGES_TO_AVERAGE" {
                      w831 = Register_name."AVG_CONTROL"  # Register name
                      w837 = TRUE  # Write/Read  (Get=true)
                      n221 = call "Set or Get SPI Register_3.vi"("Write/Read (Get=true)"=w837, "error in (no error)"=w834, "Register name"=w830, "port"=w835, "Handle"=w836) -> ("error out"=w832:errorcluster, "Read Data (16 bit)"=w827:u16, "port out"=w828:u8, "handle out"=w829:u16)  [unwired: 3 in]
                      n222 = local write "*Averaging in HW"(w827) -> ()
                    }
                    frame "AVG_CONTROL" {
                      w847 = Register_name."SPECTROMETER SN"  # Register name
                      w853 = TRUE  # Write/Read  (Get=true)
                      n223 = call "Set or Get SPI Register_3.vi"("Write/Read (Get=true)"=w853, "error in (no error)"=w850, "Register name"=w846, "port"=w851, "Handle"=w852) -> ("error out"=w848:errorcluster, "Read Data (16 bit)"=w843:u16, "port out"=w844:u8, "handle out"=w845:u16)  [unwired: 3 in]
                      n224 = Number To Boolean Array(number=w843) -> (Boolean array=w842:bool[])
                      n225 = Index Array(array=w842, index #1=0 ("index"), index #2=1 ("index")) -> (element #1=w839:bool, element #2=w838:bool)
                      n226 = local write "*Auto trig"(w839) -> ()
                      n227 = local write "Average in progress"(w838) -> ()
                    }
                    frame "SPECTROMETER SN" {
                      w858 = Register_name."SKIPPING_START"  # Register name
                      w864 = TRUE  # Write/Read  (Get=true)
                      n228 = call "Set or Get SPI Register_3.vi"("Write/Read (Get=true)"=w864, "error in (no error)"=w861, "Register name"=w857, "port"=w862, "Handle"=w863) -> ("error out"=w859:errorcluster, "Read Data (16 bit)"=w854:u16, "port out"=w855:u8, "handle out"=w856:u16)  [unwired: 3 in]
                      n229 = local write "*Spectrometer SN"(w854) -> ()
                    }
                    frame "SKIPPING_START" {
                      w869 = Register_name."SKIPPING_END"  # Register name
                      w875 = TRUE  # Write/Read  (Get=true)
                      n230 = call "Set or Get SPI Register_3.vi"("Write/Read (Get=true)"=w875, "error in (no error)"=w872, "Register name"=w868, "port"=w873, "Handle"=w874) -> ("error out"=w870:errorcluster, "Read Data (16 bit)"=w865:u16, "port out"=w866:u8, "handle out"=w867:u16)  [unwired: 3 in]
                      n231 = local write "Skipping start read buffer"(w865) -> ()
                      n232 = local write "*First pixel of interest"(w865) -> ()
                    }
                    frame "SKIPPING_END" {
                      w880 = Register_name."debug"  # Register name
                      w886 = TRUE  # Write/Read  (Get=true)
                      n233 = call "Set or Get SPI Register_3.vi"("Write/Read (Get=true)"=w886, "error in (no error)"=w883, "Register name"=w879, "port"=w884, "Handle"=w885) -> ("error out"=w881:errorcluster, "Read Data (16 bit)"=w876:u16, "port out"=w877:u8, "handle out"=w878:u16)  [unwired: 3 in]
                      n234 = local write "Skipping end read buffer"(w876) -> ()
                      n235 = local write "*Last pixel of interest"(w876) -> ()
                    }
                    frame "debug" {
                      w891 = Register_name."Production mode"  # Register name
                      w897 = TRUE  # Write/Read  (Get=true)
                      n236 = call "Set or Get SPI Register_3.vi"("Write/Read (Get=true)"=w897, "error in (no error)"=w894, "Register name"=w890, "port"=w895, "Handle"=w896) -> ("error out"=w892:errorcluster, "Read Data (16 bit)"=→"Debug":u16, "port out"=w888:u8, "handle out"=w889:u16)  [unwired: 3 in]
                    }
                    frame "Production mode" {
                      w908 = TRUE  # Write/Read  (Get=true)
                      n237 = call "Set or Get SPI Register_3.vi"("Write/Read (Get=true)"=w908, "error in (no error)"=w905, "Register name"=w902, "port"=w906, "Handle"=w907) -> ("error out"=w903:errorcluster, "Read Data (16 bit)"=w899:u16, "port out"=w900:u8, "handle out"=w901:u16)  [unwired: 3 in]
                      n238 = local write "*Production mode"(w899) -> ()
                    }
                  }
                  n239 = local read "Skipping start read buffer"() -> (w600:u16)
                  n240 = local read "Skipping end read buffer"() -> (w599:u16)
                  n241 = Or(x=w602, y=w605) -> (x .or. y?=w601:bool)
                }
                n242 = Equal To 0?(x=w534) -> (x = 0?=w544:bool)
                n243 = Equal To 0?(x=w533) -> (x = 0?=w545:bool)
                n244 = call "Get Calib data.vi"("error in (no error)"=w538, "port"=w537, "Handle"=w536) -> ("error out"=w535:errorcluster, "Cal coef"=w539:dbl[], "port out"=w529:u8, "handle out"=w530:u16)  [unwired: 4 in]
                n245 = stacked-sequence {
                  tunnel: w535 -> [_ _ _ w573 _ _]
                  tunnel: [_ _ _ w573 _ _] -> w527
                  tunnel: [_ _ _ w572 _ _] -> w528
                  frame #0 {
                    # "Only CCD supports MPP"
                    n246 = local read "*Detector type"() -> (w551:u16)
                    n247 = case shown="0, Default" w551 {
                      frame 0, Default {
                        # "CMOS-type"
                        n248 = property on="*MPP mode change" class="DigNum (strict)"("DisabledEnum"=T9."Disabled and Grayed Out" ("Disabled")) -> ()  [unwired: 2 in, 2 out]
                      }
                      frame 1 {
                        # "CCD type S11156"
                        n249 = property on="*MPP mode change" class="DigNum (strict)"("DisabledEnum"=T9."Enabled" ("Disabled")) -> ()  [unwired: 2 in, 2 out]
                      }
                    }
                  }
                  frame #1 {
                    # "Time per clock: Slow CMOS?"
                    n250 = local read "*Detector type"() -> (w559:u16)
                    n251 = local read "*FW - Variant"() -> (w558:u16)
                    n252 = Equal To 0?(x=w559) -> (x = 0?=w555:bool)
                    n253 = Equal?(x=w558, y=u16 2) -> (x = y?=w556:bool)
                    n254 = And(x=w555, y=w556) -> (x .and. y?=w554:bool)
                    n255 = case shown="False" w554 {
                      frame False {
                        # "Full speed for everything else\nUnless slowed down again..."
                        n256 = local write "SPI clock frequency [Hz]"(u32 24000000 ("SPI clock frequency [Hz]")) -> ()
                      }
                      frame True {
                        n257 = local write "msPerClock"(0.001 ("msPerClock")) -> ()
                        n258 = local write "SPI clock frequency [Hz]"(u32 4800000 ("SPI clock frequency [Hz]")) -> ()
                      }
                    }
                  }
                  frame #2 {
                    # "Time per clock: Slow CCD?"
                    n259 = local read "*Detector type"() -> (w564:u16)
                    n260 = local read "*FW - Variant"() -> (w569:u16)
                    n261 = Equal?(x=u16 1 ("y"), y=w564) -> (x = y?=w563:bool)
                    n262 = Equal?(x=w569, y=u16 1) -> (x = y?=w566:bool)
                    n263 = And(x=w563, y=w566) -> (x .and. y?=w567:bool)
                    n264 = case shown="False" w567 {
                      frame False {
                      }
                      frame True {
                        n265 = local write "msPerClock"(0.0004 ("msPerClock")) -> ()
                        n266 = local write "SPI clock frequency [Hz]"(u32 12000000 ("SPI clock frequency [Hz]")) -> ()
                      }
                    }
                  }
                  frame #3 {
                    # "Set SPI speed"
                    n267 = local read "SPI clock frequency [Hz]"() -> (w572:u32)
                  }
                  frame #4 {
                    # "Premium features: DISB-101S"
                    n268 = local read "*Detector type"() -> (w579:u16)
                    n269 = local read "*FW - Variant"() -> (w578:u16)
                    n270 = Equal To 0?(x=w579) -> (x = 0?=w575:bool)
                    n271 = Equal?(x=w578, y=u16 1) -> (x = y?=w576:bool)
                    n272 = And(x=w575, y=w576) -> (x .and. y?=w574:bool)
                    n273 = case shown="False" w574 {
                      frame False {
                      }
                      frame True {
                        n274 = property on="*First pixel of interest" class="DigNum (strict)"("DisabledEnum"=T9."Enabled" ("Disabled")) -> ()  [unwired: 2 in, 2 out]
                        n275 = property on="*Last pixel of interest" class="DigNum (strict)"("DisabledEnum"=T9."Enabled" ("Disabled")) -> ()  [unwired: 2 in, 2 out]
                      }
                    }
                  }
                  frame #5 {
                  }
                }
                n276 = And(x=w544, y=w545) -> (x .and. y?=w546:bool)
                n277 = stacked-sequence {
                  tunnel: w539 -> [w595]
                  tunnel: [w593] -> w542
                  tunnel: [w592] -> w540
                  tunnel: w532 -> [_]
                  frame #0 {
                    n278 = local read "*Pixels per image"() -> (w594:u16)
                    n279 = for {
                      N: w594 -> [_]
                      tunnel: w595 -> [w598]
                      tunnel: [w597] -> w592 mode=indexing
                      tunnel: [w596] -> w593 mode=indexing
                      i -> [w596]
                      n280 = call "Pix_lamda_Poly_conversion.vi"("Pixels"=w596, "Cal coef"=w598) -> ("Lamda(nm)"=w597:dbl)  [unwired: 7 in, 6 out]
                    }
                  }
                }
                n281 = local write "*Cal coef"(w539) -> ()
                n282 = case shown="True" w546 {
                  tunnel: w540 -> [w589 w590]
                  tunnel: [w587 w590] -> w541
                  tunnel: w542 -> [w585 w591]
                  tunnel: [w584 w591] -> w543
                  tunnel: w533 -> [w583 _]
                  tunnel: w534 -> [w582 _]
                  frame False {
                    n283 = Subtract(x=w583, y=w582) -> (x-y=w588:u16)
                    n284 = Increment(x=w588) -> (x+1=w586:u16)
                    n285 = Array Subset(array=w589, index=w582, length=w586) -> (w587:dbl[])
                    n286 = Array Subset(array=w585, index=w582, length=w586) -> (w584:i32[])
                  }
                  frame True {
                  }
                }
                n287 = local write "*Wavelength axis"(w541) -> ()
                n288 = call "Spi_Set Frequency.vi"("error in (no error)"=w527, "Frequency"=w528, "port"=w529, "Handle"=w530) -> ("Actual frequency"=w531:u32)  [unwired: 4 in, 3 out]
                n289 = local write "SPI clock frequency [Hz]"(w531) -> ()
                n290 = local write "Pixel axis"(w543) -> ()
              }
              frame #2 {
                # "take dark scan, save to file, or zero dark scan"
                n291 = local read "Get Dark?"() -> (w911:bool)
                n292 = case shown="False" w911 {
                  tunnel: [w922 w929] -> w912
                  tunnel: [w914 "Zero Dark LIBS"] -> w909
                  tunnel: w910 -> [w915 w930]
                  frame True {
                    n293 = Format Date/Time String(time format string (%c)="%y%m%d%H%M%S") -> (date/time string=w919:string)  [unwired: 2 in]
                    n294 = Concatenate Strings(w919, "LIBS" ("string"), "Dark" ("string")) -> (w921:string)
                    n295 = Build Path(base path=path "C:/Program Files (x86)/National Instruments/LabVIEW 2019/instr.lib/LPT/DataLIBS", name or relative path=w921) -> (appended path=w925:path)
                    n296 = call "LPT-LIBS-Spectra Acquire.vi"("error in"=w915) -> ("error out"=w923:errorcluster, "Raw Data"=w914:dbl[])  [unwired: 7 in, 2 out]
                    n297 = call-poly <vilib>:"Write Delimited Spreadsheet.vi"("file path (dialog if empty)"=w925, "1D data"=w914, "error in (no error)"=w923, "transpose? (no:F)"=TRUE) -> ("error out"=w922:errorcluster)  [unwired: 10 in, 1 out]
                  }
                  frame False {
                    n298 = local read "Start"() -> (w928:bool)
                    n299 = call "LPT-FileSave.vi"("error in (no error)"=w930, "Data\\Dark"=FALSE ("Data\\Dark"), "Raman\\LIBS"=w928, "Array"="Zero Dark LIBS") -> ("error out"=w929:errorcluster)  [unwired: 7 in]
                  }
                }
                "LIBS Dark Spectra" <- w909
                n300 = case shown="False" w911 {
                  frame False {
                  }
                  frame True {
                    n301 = local write "STATUS"("Getting Dark Spectrum") -> ()
                  }
                }
              }
              frame #3 {
                # "set power, verify power, auto focus"
                n302 = case shown="True" "Auto Set\nLaser Frequency" {
                  tunnel: w936 -> [w1017 w1019]
                  tunnel: [w1016 w1018] -> w934
                  frame False {
                    n303 = call "labview dds-3x25 LPT.vi"("error in (no error)"=w1017, "Frequency"="LIBS Laser Frequency (Hz)") -> ("error out"=w1016:errorcluster)  [unwired: 1 in]
                    n304 = Number To Decimal String(number="LIBS Laser Frequency (Hz)") -> (decimal integer string=w1013:string)  [unwired: 1 in]
                    n305 = Concatenate Strings("Setting LIBS Laser Frequency to ", w1013) -> (w1015:string)
                    n306 = local write "STATUS"(w1015) -> ()
                  }
                  frame True {
                    n307 = while {
                      tunnel: w1019 -> [w1022]
                      tunnel: [w1032] -> w1018
                      i -> [w1026]
                      stop <- w1023 stop-if-true
                      n308 = local read "LIBS Dark Spectra"() -> (w1034:dbl[])
                      n309 = Multiply(x=w1026, y=90) -> (x*y=w1020:i32)
                      n310 = call "labview dds-3x25 LPT.vi"("error in (no error)"=w1022, "Frequency"=w1020) -> ("error out"=w1021:errorcluster)  [unwired: 1 in]
                      n311 = Equal?(x=w1026, y=10) -> (x = y?=w1024:bool)
                      n312 = call "LPT-LIBS-Spectra Acquire.vi"("error in"=w1021, "LIBS Dark Array"=w1034) -> ("error out"=w1032:errorcluster, "Raw Data"=w1033:dbl[])  [unwired: 6 in, 2 out]
                      n313 = case shown="True" w1024 {
                        frame False {
                        }
                        frame True {
                          n314 = One Button Dialog(message="No/Poor signal") -> ()  [unwired: 1 in, 1 out]
                        }
                      }
                      n315 = Array Max & Min(array=w1033) -> (max value=w1028:dbl)  [unwired: 3 out]
                      n316 = local write "STATUS"("Auto Setting Laser Frequency") -> ()
                      n317 = Greater?(x=w1028, y=3000.0) -> (0:w1029:bool)
                      n318 = Or(x=w1029, y=w1024) -> (x .or. y?=w1023:bool)
                    }
                  }
                }
                n319 = local read "AUT FOCUS"() -> (w935:bool)
                n320 = case shown="False" FALSE {
                  tunnel: w935 -> [_ w982]
                  tunnel: w934 -> [w938 w981]
                  tunnel: [w937 w980] -> w933
                  frame False {
                    n321 = stacked-sequence {
                      seq-local: [w941 _ _] -> [_ w969 _]
                      seq-local: [w940 _ _] -> [_ w972 _]
                      seq-local: ["STAGE START 2" _ _] -> [_ w973 _]
                      tunnel: [w943 _ _] -> w937
                      tunnel: w938 -> [w943 _ _]
                      frame #0 {
                        n322 = Subtract(x="STAGE STOP 2", y="STAGE START 2") -> (x-y=w945:i32)
                        n323 = Divide(x=w945, y="#of steps 3") -> (x/y=w940:dbl)
                        n324 = Increment(x="#of steps 3") -> (x+1=w946:i32)
                        n325 = for {
                          N: w946 -> [_]
                          tunnel: w940 -> [w956]
                          tunnel: "STAGE START 2" -> [w952]
                          shift-right: [w948] -> w941
                          shift-left: sgl[] [] -> [w949]
                          i -> [w955]
                          n326 = stacked-sequence {
                            tunnel: [_ w958] -> w950
                            frame #0 {
                              n327 = Wait (ms)(milliseconds to wait=u32 1000) -> ()  [unwired: 1 out]
                            }
                            frame #1 {
                              n328 = call "LPT-SpectraWiz-Acquire W Dark.vi"() -> ("Buffer"=w958:sgl[])  [unwired: 10 in, 1 out]
                            }
                          }
                          "Raw Data 2" <- w950
                          n329 = Multiply(x=w956, y=w955) -> (x*y=w954:dbl)
                          n330 = Add(x=w952, y=w954) -> (x+y=w953:dbl)
                          n331 = stacked-sequence {
                            tunnel: w953 -> [w961 _ _]
                            frame #0 {
                              n332 = Number To Decimal String(number=w961) -> (decimal integer string=w960:string)  [unwired: 1 in]
                              "NUMBER 2" <- w960
                              n333 = Concatenate Strings("MOV ", w960) -> (→"COMMAND 3":string)
                              "Position (um) 2" <- w961
                            }
                            frame #1 {
                              n334 = local read "COMMAND 3"() -> (w967:string)
                              n335 = call "Serial Write and Read on Two Ports 3.0.vi"("Write String"=w967) -> ("Read String"=w966:string)  [unwired: 10 in]
                              "COMMAND1 READ 3" <- w966
                              n336 = local read "NUMBER 2"() -> (w965:string)
                              n337 = Match Pattern(string=w966, regular expression=w965) -> (match substring=w964:string)  [unwired: 1 in, 3 out]
                              n338 = Equal?(x=w964, y=w965) -> (x = y?=→"AUT FOCUS STATUS 2":bool)
                            }
                            frame #2 {
                              n339 = Wait (ms)(milliseconds to wait=u32 100) -> ()  [unwired: 1 out]
                            }
                          }
                          n340 = Add Array Elements(numeric array=w950) -> (sum=w951:sgl)
                          "power sum 2" <- w951
                          n341 = Build Array (concatenate)(w949, w951) -> (w948:sgl[])
                        }
                      }
                      frame #1 {
                        (unwired) 10.0 ("Position (mm)")
                        (unwired) 500.0 ("MaxPosition")
                        (unwired) sgl 3651732.0 ("max value")
                        n342 = Array Max & Min(array=w969) -> (max value=w971:sgl, max index (indices)=w975:i32)  [unwired: 2 out]
                        n343 = Multiply(x=w975, y=w972) -> (x*y=w974:dbl)
                        n344 = local write "max value"(w971) -> ()
                        n345 = Add(x=w974, y=w973) -> (x+y=w970:dbl)
                        n346 = local write "Position (um) 2"(w970) -> ()
                        n347 = local write "MaxPosition"(w970) -> ()
                      }
                      frame #2 {
                        n348 = local read "Position (um) 2"() -> (w977:dbl)
                        n349 = Number To Decimal String(number=w977) -> (decimal integer string=w978:string)  [unwired: 1 in]
                        n350 = Concatenate Strings("MOV ", w978) -> (w976:string)
                        n351 = call "Serial Write and Read on Two Ports 3.0.vi"("Write String"=w976) -> ()  [unwired: 10 in, 1 out]
                      }
                    }
                  }
                  frame True {
                    n352 = case shown="True" w982 {
                      tunnel: w981 -> [w983 w993]
                      tunnel: [w983 w984] -> w980
                      frame False {
                      }
                      frame True {
                        n353 = local read "LED 1 STATUS"() -> (w986:bool)
                        n354 = local read "Set End Position (um)"() -> (w990:dbl)
                        n355 = case shown="True" w986 {
                          tunnel: w990 -> [_ w1006]
                          tunnel: [w998 w1003] -> w989
                          tunnel: [w997 10] -> w988
                          tunnel: [w996 w1002] -> w987
                          frame False {
                            n356 = local read "#of steps A"() -> (w997:i32)
                            n357 = local read "STAGE STOP A"() -> (w996:i32)
                            n358 = local read "STAGE START A"() -> (w998:i32)
                          }
                          frame True {
                            n359 = Subtract(x=w1006, y=1) -> (x-y=w999:dbl)
                            n360 = Less?(x=w999, y=1) -> (x < y?=w1001:bool)
                            n361 = case shown="False" w1001 {
                              tunnel: w999 -> [w1008 _]
                              tunnel: [w1008 1] -> w1003
                              tunnel: [w1007 3] -> w1002
                              frame False {
                                n362 = Add(x=2, y=w1008) -> (x+y=w1007:dbl)
                              }
                              frame True {
                              }
                            }
                          }
                        }
                        n363 = local read "LIBS Dark Spectra"() -> (w991:dbl[])
                        n364 = call "LPT-Actuonix-LIBS-AutoFocus.vi"("LIBS Dark Array"=w991, "error in (no error)"=w993, "STOP"=w987, "START"=w989, "#of steps"=w988) -> ("error out"=w985:errorcluster, "Position (mm)"=w992:dbl)  [unwired: 2 in, 3 out]
                        n365 = local write "Set End Position (um)"(w992) -> ()
                        n366 = in-place {
                          in-place-border: w985 -> [w995]
                          in-place-border: [w995] -> w984
                          n367 = local write "LED 1 STATUS"(TRUE) -> ()
                        }
                      }
                    }
                  }
                }
                n368 = case shown="True" w935 {
                  frame False {
                  }
                  frame True {
                    n369 = local write "STATUS"("Autofocus") -> ()
                  }
                }
              }
            }
            n370 = local read "AutoAcquire"() -> (w357:bool)
            n371 = case shown="True" w357 {
              tunnel: [w386 w398] -> w349
              tunnel: w362 -> [w383 w397]
              frame True {
                n372 = local read "Number of Scans \nto Auto Acquire"() -> (w384:i32)
                n373 = call "LPT-ImageSnapandSave.vi"("error in"=w383, "Raman\\LIBS"=FALSE ("Raman\\LIBS")) -> ("error out"=w382:errorcluster)  [unwired: 9 in]
                n374 = for {
                  N: w384 -> [_]
                  shift-right: [w391] -> w386
                  shift-left: w382 -> [w389]
                  w393 = FALSE ("Raman\\LIBS")
                  n375 = local read "LIBS Dark Spectra"() -> (w387:dbl[])
                  n376 = call "LPT-LIBS-Spectra Acquire.vi"("error in"=w389, "LIBS Dark Array"=w387) -> ("error out"=w395:errorcluster, "Removed background"=→"Removed background":dbl[], "Raw Data"=w396:dbl[], "Spectrum"=w390:cluster{dbl[], dbl[]})  [unwired: 6 in]
                  n377 = local write "Spectrum"(w390) -> ()
                  n378 = call "LPT-FileSave.vi"("error in (no error)"=w395, "Data\\Dark"=TRUE ("Data\\Dark"), "Raman\\LIBS"=w393, "Array"=w396) -> ("error out"=w392:errorcluster)  [unwired: 7 in]
                  n379 = call "LPT-XYFileSave.vi"("error in (no error)"=w392, "Raman\\LIBS"=w393, "Spectrum"=w390) -> ("error out"=w391:errorcluster)  [unwired: 8 in]
                }
                n380 = local write "STATUS"("Aquiring Spectrum" ("STATUS")) -> ()
              }
              frame False {
                n381 = while {
                  tunnel: [w400] -> w398
                  tunnel: w397 -> [w401]
                  stop <- w399 stop-if-true
                  n382 = local read "INTERACTIVE CONTROLS"() -> (w402:T2)
                  n383 = case shown="\"ReFocus\"" w402 {
                    tunnel: w401 -> [w411 w422 w443 w466 w477 w483 w500]
                    tunnel: [w412 w420 w441 w464 w476 w481 w499] -> w400
                    frame "Acquire" {
                      n384 = call "LPT-ImageSnapandSave.vi"("error in"=w411, "Raman\\LIBS"=FALSE) -> ("error out"=w409:errorcluster)  [unwired: 9 in]
                      n385 = local read "LIBS Dark Spectra"() -> (w417:dbl[])
                      n386 = call "LPT-LIBS-Spectra Acquire.vi"("error in"=w409, "LIBS Dark Array"=w417) -> ("error out"=w415:errorcluster, "Removed background"=w408:dbl[], "Raw Data"=w416:dbl[], "Spectrum"=w405:cluster{dbl[], dbl[]})  [unwired: 6 in]
                      n387 = local write "Removed background"(w408) -> ()
                      n388 = local write "Spectrum"(w405) -> ()
                      n389 = call "LPT-FileSave.vi"("error in (no error)"=w415, "Data\\Dark"=TRUE ("Data\\Dark"), "Raman\\LIBS"=FALSE ("Raman\\LIBS"), "Array"=w416) -> ("error out"=w407:errorcluster)  [unwired: 7 in]
                      n390 = call "LPT-XYFileSave.vi"("error in (no error)"=w407, "Raman\\LIBS"=FALSE, "Spectrum"=w405) -> ("error out"=w406:errorcluster)  [unwired: 8 in]
                      n391 = flat-sequence {
                        tunnel: w406 -> [w418]
                        tunnel: [w418] -> w412
                        frame #0 {
                          n392 = Wait (ms)(milliseconds to wait=1000) -> ()  [unwired: 1 out]
                        }
                      }
                    }
                    frame "ReFocus" {
                      n393 = local read "Set End Position (um)"() -> (w430:dbl)
                      n394 = Subtract(x=w430, y=1) -> (x-y=w426:dbl)
                      n395 = Less?(x=w426, y=1) -> (x < y?=w427:bool)
                      n396 = case shown="False" w427 {
                        tunnel: [w438 1] -> w428
                        tunnel: [w437 3] -> w429
                        tunnel: w426 -> [w438 _]
                        frame False {
                          n397 = Add(x=2, y=w438) -> (x+y=w437:dbl)
                        }
                        frame True {
                        }
                      }
                      n398 = local read "LIBS Dark Spectra"() -> (w431:dbl[])
                      n399 = call "LPT-Actuonix-LIBS-AutoFocus.vi"("LIBS Dark Array"=w431, "error in (no error)"=w422, "STOP"=w429, "START"=w428, "#of steps"=10) -> ("error out"=w421:errorcluster, "Position (mm)"=w432:dbl)  [unwired: 2 in, 3 out]
                      n400 = local write "Set End Position (um)"(w432) -> ()
                      n401 = flat-sequence {
                        tunnel: w421 -> [w434]
                        tunnel: [w434] -> _
                        tunnel: [w434] -> w420
                        frame #0 {
                          n402 = local write "INTERACTIVE CONTROLS"(6) -> ()
                          n403 = Wait (ms)(milliseconds to wait=1000) -> ()  [unwired: 1 out]
                        }
                      }
                    }
                    frame "ReSet Power" {
                      n404 = while {
                        tunnel: [w459] -> w442
                        tunnel: w443 -> [w453]
                        i -> [w450]
                        stop <- w454 stop-if-true
                        n405 = local read "power setting from LQ"() -> (w458:string)
                        n406 = Multiply(x=w450, y=100) -> (x*y=w448:i32)
                        n407 = local read "LIBS Dark Spectra"() -> (w462:dbl[])
                        n408 = Equal?(x=w450, y=10) -> (x = y?=w447:bool)
                        n409 = call "LPT-LIBS-Burst Mod.vi"("Delay (50ms)"=50, "Frequency (10 Hz)"=w448, "error in (no error)"=w453, "VISA resource name"=w458) -> ("error out"=w461:errorcluster)  [unwired: 6 in, 1 out]
                        n410 = case shown="True" w447 {
                          frame False {
                          }
                          frame True {
                            n411 = One Button Dialog(message="No/Poor signal") -> ()  [unwired: 1 in, 1 out]
                          }
                        }
                        n412 = call "LPT-LIBS-Spectra Acquire.vi"("error in"=w461, "LIBS Dark Array"=w462) -> ("error out"=w459:errorcluster, "Raw Data"=w460:dbl[])  [unwired: 6 in, 2 out]
                        n413 = Array Max & Min(array=w460) -> (max value=w455:dbl)  [unwired: 3 out]
                        n414 = Greater?(x=w455, y=3000.0) -> (0:w457:bool)
                        n415 = Or(x=w457, y=w447) -> (x .or. y?=w454:bool)
                      }
                      n416 = flat-sequence {
                        tunnel: [w444] -> w441
                        tunnel: w442 -> [w444]
                        frame #0 {
                          n417 = local write "INTERACTIVE CONTROLS"(6) -> ()
                          n418 = Wait (ms)(milliseconds to wait=1000) -> ()  [unwired: 1 out]
                        }
                      }
                    }
                    frame "New Dark" {
                      n419 = stacked-sequence {
                        tunnel: w466 -> [w473]
                        tunnel: [w474] -> w465
                        frame #0 {
                          n420 = call "LPT-SpectraWiz-GetDark.vi"("error in"=w473) -> ("error out"=w475:errorcluster, "Dark Spectra"=w470:sgl[])  [unwired: 9 in]
                          n421 = local write "LIBS Dark Spectra"(w470) -> ()
                          n422 = call "LPT-FileSave.vi"("error in (no error)"=w475, "Data\\Dark"=FALSE ("Data\\Dark"), "Raman\\LIBS"=FALSE ("Raman\\LIBS"), "Array"=w470) -> ("error out"=w474:errorcluster)  [unwired: 7 in]
                        }
                      }
                      n423 = flat-sequence {
                        tunnel: w465 -> [w468]
                        tunnel: [w468] -> w464
                        frame #0 {
                          n424 = local write "INTERACTIVE CONTROLS"(6) -> ()
                          n425 = Wait (ms)(milliseconds to wait=1000) -> ()  [unwired: 1 out]
                        }
                      }
                    }
                    frame "Parameter Reset" {
                      n426 = flat-sequence {
                        tunnel: w477 -> [w478]
                        tunnel: [w478] -> w476
                        frame #0 {
                          n427 = local write "INTERACTIVE CONTROLS"(6) -> ()
                          n428 = Wait (ms)(milliseconds to wait=500) -> ()  [unwired: 1 out]
                        }
                      }
                    }
                    frame "Material ID" {
                      n429 = local read "Analysis Program"() -> (w484:T3)
                      n430 = case shown="\"Atom Analyzer\", Default" w484 {
                        tunnel: w483 -> [w489 w492 w497]
                        tunnel: [w487 w491 w496] -> w482
                        frame "Atom Analyzer", Default {
                          n431 = call <vilib>:"System Exec.vi"("wait until completion? (T)"=TRUE, "error in (no error)"=w489, "command line"="C:\\Users\\Raman\\Desktop\\AtomAnalyzer_202011.00_Windows\\AtomAnalyzer\\bin\\AtomAnalyzer.exe") -> ("error out"=w487:errorcluster)  [unwired: 5 in, 3 out]
                        }
                        frame "Spectra Gryph" {
                          n432 = call <vilib>:"System Exec.vi"("wait until completion? (T)"=TRUE, "error in (no error)"=w492, "command line"="C:\\Program Files (x86)\\Spectragryph 1.2\\SpectraGryph.exe" ("standard input")) -> ("error out"=w491:errorcluster)  [unwired: 5 in, 3 out]
                        }
                        frame "Know It All" {
                          n433 = call <vilib>:"System Exec.vi"("wait until completion? (T)"=TRUE, "error in (no error)"=w497, "command line"="C:\\Program Files\\KnowItAll\\Bin\\KnowItAll.exe") -> ("error out"=w496:errorcluster)  [unwired: 5 in, 3 out]
                        }
                      }
                      n434 = flat-sequence {
                        tunnel: w482 -> [w485]
                        tunnel: [w485] -> w481
                        frame #0 {
                          n435 = local write "INTERACTIVE CONTROLS"(6) -> ()
                        }
                      }
                    }
                    frame "Do Nothing", Default {
                      n436 = flat-sequence {
                        tunnel: w500 -> [w501]
                        tunnel: [w501] -> _
                        tunnel: [w501] -> w499
                        frame #0 {
                          n437 = Wait (ms)(milliseconds to wait=500) -> ()  [unwired: 1 out]
                        }
                      }
                    }
                  }
                  n438 = local read "EXIT INTERACTIVE CONTROL"() -> (w399:bool)
                  n439 = local write "STATUS"("Click an Interactive Control or EXIT INT CNTL to Exit" ("STATUS")) -> ()
                }
              }
            }
            n440 = flat-sequence {
              tunnel: w349 -> [w363]
              tunnel: [w363] -> w348
              frame #0 {
                n441 = local write "INTERACTIVE CONTROLS"(6) -> ()
              }
            }
            n442 = local read "ID spectra"() -> (w358:bool)
            n443 = case shown="True" w358 {
              tunnel: w351 -> [_ w370]
              frame False {
              }
              frame True {
                n444 = local read "Analysis Program"() -> (w371:T3)
                n445 = case shown="\"Know It All\"" w371 {
                  tunnel: w370 -> [w372 w377 w380]
                  frame "Atom Analyzer", Default {
                    n446 = call <vilib>:"System Exec.vi"("wait until completion? (T)"=TRUE, "error in (no error)"=w372, "command line"="C:\\Users\\Raman\\Desktop\\AtomAnalyzer_202011.00_Windows\\AtomAnalyzer\\bin\\AtomAnalyzer.exe" ("standard input")) -> ()  [unwired: 5 in, 4 out]
                  }
                  frame "Spectra Gryph" {
                    n447 = call <vilib>:"System Exec.vi"("wait until completion? (T)"=TRUE, "error in (no error)"=w377, "command line"="C:\\Program Files (x86)\\Spectragryph 1.2\\SpectraGryph.exe" ("standard input")) -> ()  [unwired: 5 in, 4 out]
                  }
                  frame "Know It All" {
                    n448 = call <vilib>:"System Exec.vi"("wait until completion? (T)"=TRUE, "error in (no error)"=w380, "command line"="C:\\Program Files\\KnowItAll\\Bin\\KnowItAll.exe" ("standard input")) -> ()  [unwired: 5 in, 4 out]
                  }
                }
              }
            }
            n449 = call "labview dds-3x25 LPT.vi"("error in (no error)"=w348, "Frequency"=0) -> ("error out"=w352:errorcluster)  [unwired: 1 in]
            n450 = flat-sequence {
              tunnel: [TRUE] -> w353
              tunnel: w352 -> [w366]
              tunnel: [w366] -> w351
              frame #0 {
                n451 = local write "EXIT INTERACTIVE CONTROL"(FALSE) -> ()
                n452 = local write "Start"(FALSE) -> ()
                n453 = local write "STATUS"("Acquisition Complete - Ready to Acquire") -> ()
              }
            }
          }
        }
      }
    }
  }
  n454 = while {
    stop <- TRUE continue-if-true
    n455 = stacked-sequence {
      frame #0 {
        n456 = Wait (ms)(milliseconds to wait=u32 10) -> ()  [unwired: 1 out]
      }
      frame #1 {
        w1039 = FALSE ("LED 2")
        n457 = feedback #1(w1039) -> (w1047:bool)
        n458 = Equal?(x="LED 1", y=w1047) -> (x = y?=w1044:bool)
        n459 = feedback-in #1("LED 1") -> ()
        n460 = feedback #2(w1039) -> (w1046:bool)
        n461 = Equal?(x="LED 2", y=w1046) -> (x = y?=w1043:bool)
        n462 = feedback-in #2("LED 2") -> ()
        n463 = case shown="False" w1043 {
          tunnel: "LED 2" -> [w1054 _]
          frame False {
            n464 = case shown="True" w1054 {
              tunnel: ["LED2 OFF" "LED2 ON"] -> w1053
              frame False {
              }
              frame True {
              }
            }
            n465 = local write "COMMAND 1"(w1053) -> ()
          }
          frame True {
          }
        }
        n466 = case shown="False" w1044 {
          tunnel: "LED 1" -> [w1058 _]
          frame False {
            n467 = case shown="True" w1058 {
              tunnel: ["LED1 OFF" "LED1 ON"] -> w1057
              frame False {
              }
              frame True {
              }
            }
            n468 = local write "COMMAND 1"(w1057) -> ()
          }
          frame True {
          }
        }
        n469 = Not(x=w1044) -> (.not. x?=w1041:bool)
        n470 = Not(x=w1043) -> (.not. x?=w1042:bool)
        n471 = Compound Arithmetic op=OR(w1041, w1042) -> (w1040:bool)
        n472 = stacked-sequence {
          tunnel: w1040 -> [w1049]
          frame #0 {
            n473 = case shown="True" w1049 {
              frame False {
              }
              frame True {
                n474 = call "Serial Write and Read on Two Ports 3.0.vi"("VISA Resource (write)"="LED Resource (write)", "Write String"="COMMAND 1") -> ("Read String"=→"COMMAND1 READ":string)  [unwired: 9 in]
              }
            }
          }
        }
      }
      frame #2 {
        w1065 = "LED2 OFF" ("y")
        w1064 = "LED2 ON" ("y")
        w1063 = "LED1 OFF" ("y")
        w1062 = "LED1 ON" ("y")
        n475 = local read "COMMAND1 READ"() -> (w1061:string)
        n476 = Match Pattern(string=w1061, regular expression=w1065) -> (match substring=w1070:string)  [unwired: 1 in, 3 out]
        n477 = Match Pattern(string=w1061, regular expression=w1064) -> (match substring=w1071:string)  [unwired: 1 in, 3 out]
        n478 = Match Pattern(string=w1061, regular expression=w1063) -> (match substring=w1072:string)  [unwired: 1 in, 3 out]
        n479 = Match Pattern(string=w1061, regular expression=w1062) -> (match substring=w1073:string)  [unwired: 1 in, 3 out]
        n480 = Equal?(x=w1065, y=w1070) -> (x = y?=w1066:bool)
        n481 = Equal?(x=w1064, y=w1071) -> (x = y?=w1067:bool)
        n482 = Equal?(x=w1063, y=w1072) -> (x = y?=w1068:bool)
        n483 = Equal?(x=w1062, y=w1073) -> (x = y?=w1069:bool)
        n484 = case shown="True" w1066 {
          frame False {
          }
          frame True {
            n485 = local write "LED 2 STATUS"(FALSE ("LED 1 STATUS")) -> ()
          }
        }
        n486 = case shown="True" w1067 {
          frame False {
          }
          frame True {
            n487 = local write "LED 2 STATUS"(TRUE ("LED 1 STATUS")) -> ()
          }
        }
        n488 = case shown="True" w1068 {
          frame False {
          }
          frame True {
            n489 = local write "LED 1 STATUS"(FALSE ("LED 1 STATUS")) -> ()
          }
        }
        n490 = case shown="True" w1069 {
          frame False {
          }
          frame True {
            n491 = local write "LED 1 STATUS"(TRUE ("LED 1 STATUS")) -> ()
          }
        }
      }
      frame #3 {
        n492 = stacked-sequence {
          frame #0 {
          }
        }
      }
    }
  }
  n493 = while {
    shift-right: ["Tab Control"] -> _
    shift-left: _ -> [w1079]
    stop <- TRUE continue-if-true
    n494 = Equal?(x=w1079, y="Tab Control") -> (x = y?=w1081:bool)
    n495 = Wait (ms)(milliseconds to wait=u32 500) -> ()  [unwired: 1 out]
    n496 = local write "Camera STOP 2"(w1081) -> ()
  }
  n497 = local write "Tab Control"(w1) -> ()
  n498 = while {
    shift-right: [w1084] -> _
    shift-left: w1 -> [w1083]
    stop <- w1087 stop-if-true
    n499 = case shown="True" "START CAM TAB" {
      tunnel: [w1088 w1089] -> w1084
      tunnel: w1083 -> [_ w1089]
      frame False {
        n500 = local read "Tab Control"() -> (w1088:enum32{"Visible", "Fluorescence"})
      }
      frame True {
      }
    }
    n501 = case shown="\"Fluorescence\"" w1084 {
      frame "Fluorescence" {
        w1091 = errorcluster {"status"=FALSE, "code"=0, "source"=""} ("error in")
        n502 = call "IMAQ Create"("Image Name"="Fluorescence Cam", "error in (no error)"=w1091) -> ("New Image"=w1099:T7)  [unwired: 3 in, 1 out]
        n503 = call <vilib>:"IMAQdx Open Camera.vi"("error in"=w1091, "Session In"="Session In 2") -> ("error out"=w1093:errorcluster, "Session Out"=w1094:T1)  [unwired: 8 in]
        n504 = call <vilib>:"IMAQdx Configure Grab.vi"("error in"=w1093, "Session In"=w1094) -> ("error out"=w1096:errorcluster, "Session Out"=w1095:T1)  [unwired: 8 in]
        n505 = while {
          shift-right: [w1104] -> w1097
          shift-left: w1095 -> [w1106]
          shift-right: [w1103] -> w1098
          shift-left: w1096 -> [w1105]
          shift-right: [w1102] -> _
          shift-left: w1099 -> [w1102]
          stop <- w1100 continue-if-true
          n506 = call <vilib>:"IMAQdx Grab2.vi"("error in"=w1105, "Image In"=w1102, "Session In"=w1106) -> ("error out"=w1103:errorcluster, "Image Out"=→"Fluorescence Image":T7, "Session Out"=w1104:T1)  [unwired: 5 in, 1 out]
          n507 = Wait (ms)(milliseconds to wait=u32 10) -> ()  [unwired: 1 out]
          n508 = local read "Camera STOP 2"() -> (w1100:bool)
          n509 = local write "START CAM TAB"(w1100) -> ()
        }
        n510 = call <vilib>:"IMAQdx Close Camera.vi"("error in"=w1098, "Session In"=w1097) -> ()  [unwired: 9 in, 1 out]
      }
      frame "Visible" {
        w1115 = errorcluster {"status"=FALSE, "code"=0, "source"=""} ("error in")
        n511 = call "IMAQ Create"("Image Name"="Visible Cam", "error in (no error)"=w1115) -> ("New Image"=w1112:T7)  [unwired: 3 in, 1 out]
        n512 = call <vilib>:"IMAQdx Open Camera.vi"("error in"=w1115, "Session In"="Session In") -> ("error out"=w1113:errorcluster, "Session Out"=w1114:T1)  [unwired: 8 in]
        n513 = call <vilib>:"IMAQdx Configure Grab.vi"("error in"=w1113, "Session In"=w1114) -> ("error out"=w1110:errorcluster, "Session Out"=w1111:T1)  [unwired: 8 in]
        n514 = while {
          shift-right: [w1121] -> _
          shift-left: w1112 -> [w1121]
          shift-right: [w1120] -> w1109
          shift-left: w1111 -> [w1123]
          shift-right: [w1119] -> w1108
          shift-left: w1110 -> [w1122]
          stop <- w1118 continue-if-true
          n515 = call <vilib>:"IMAQdx Grab2.vi"("error in"=w1122, "Image In"=w1121, "Session In"=w1123) -> ("error out"=w1119:errorcluster, "Image Out"=→"Visible Image":T7, "Session Out"=w1120:T1)  [unwired: 5 in, 1 out]
          n516 = Wait (ms)(milliseconds to wait=u32 10) -> ()  [unwired: 1 out]
          n517 = local read "Camera STOP 2"() -> (w1118:bool)
          n518 = local write "START CAM TAB"(w1118) -> ()
        }
        n519 = call <vilib>:"IMAQdx Close Camera.vi"("error in"=w1108, "Session In"=w1109) -> ()  [unwired: 9 in, 1 out]
      }
    }
    n520 = Wait (ms)(milliseconds to wait=u32 10) -> ()  [unwired: 1 out]
    n521 = local read "Camera STOP"() -> (w1087:bool)
  }
  "LASER \nFOCUSED" <- FALSE ("Laser \nFocused")
  "Camera STOP" <- FALSE
  "Camera STOP 2" <- FALSE ("Camera STOP 2")
